vi "Autonomous Independent.vi"   [LabVIEW 2016]
doc: "This VI is called when autonomous begins, and will automatically be terminated when autonomous ends. You can carry out timed or sensor driven robot movement independently without needing to return to the caller."
uses:
  <vilib>/Rock Robotics/Network Tables/NT Read String.vi
panel:
  # "Be sure to right-click and choose Data Operations>>Make Current Value default if you want to save the array values with the VI"
types:
  T1 = typedef "WPI_MotorControlDeviceRef.ctl" = cluster{"DeviceStatus":errorcluster, "Type":T2, "PWM":cluster{"PWM Channel":T3, "DeadBand":T4}, "CAN":cluster{"Device Number":u8, "SetOutput VI Ref":variant, "GetOutput VI Ref":variant, "Enable VI Ref":variant, "Disable VI Ref":variant, "Data":variant}, "Invert":bool}
  T2 = typedef "WPI_MotorControlType.ctl" = enum16{"PWM", "CAN"}
  T3 = typedef "FPGA_DIOPWMChannel.ctl" = enum8{"PWM 0", "PWM 1", "PWM 2", "PWM 3", "PWM 4", "PWM 5", "PWM 6", "PWM 7", "PWM 8", "PWM 9", "PWM MXP 0", "PWM MXP 1", "PWM MXP 2", "PWM MXP 3", "PWM MXP 4", "PWM MXP 5", "PWM MXP 6", "PWM MXP 7", "PWM MXP 8", "PWM MXP 9", "Invalid"}
  T4 = typedef "WPI_PWMDeadband.ctl" = cluster{"Name":string, "maxPositivePwm":i32, "minPositivePwm":i32, "centerPwm":i32, "maxNegativePwm":i32, "minNegativePwm":i32, "angularRange":u16}
  T5 = typedef "WPI_DriverStationAllianceInfo.ctl" = enum16{"Red", "Blue", "Invalid"}
  T6 = typedef "WPI_EncoderDevRef.ctl" = cluster{"DevStatus":errorcluster, "EncoderIndex":T7, "CounterIndex":T8, "DistancePerCount":dbl, "Decoding Type":T9}
  T7 = typedef "FPGA_EncoderIdx.ctl" = enum8{"Enc 0", "Enc 1", "Enc 2", "Enc 3", "Enc 4", "Enc 5", "Enc 6", "Enc 7", "Invalid"}
  T8 = typedef "FPGA_CounterCtrSystemIndex.ctl" = enum8{"Ctr 0", "Ctr 1", "Ctr 2", "Ctr 3", "Ctr 4", "Ctr 5", "Ctr 6", "Ctr 7", "Invalid"}
  T9 = typedef "WPI_EncoderType.ctl" = enum16{"1x", "2x", "4x"}
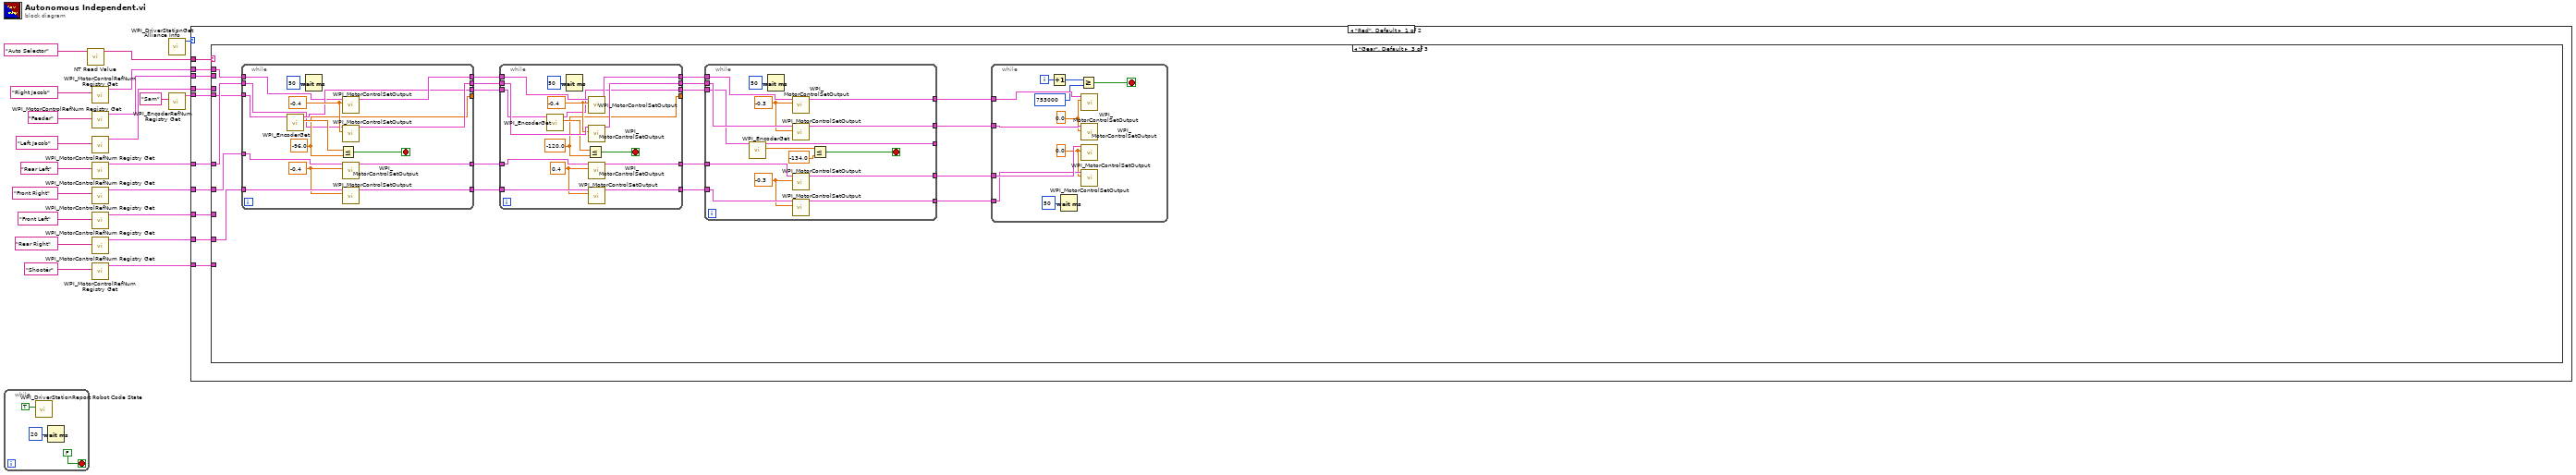
[diagram p0: block diagram]
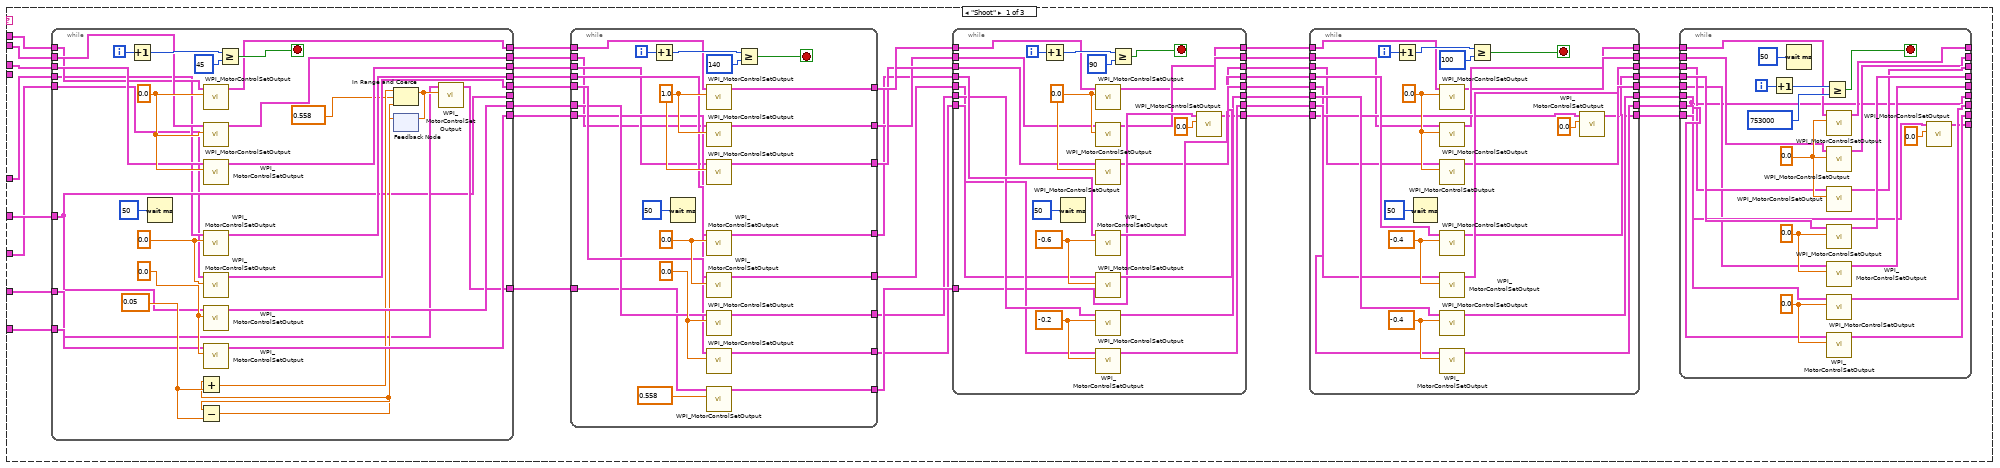
[diagram p2: hidden frame]
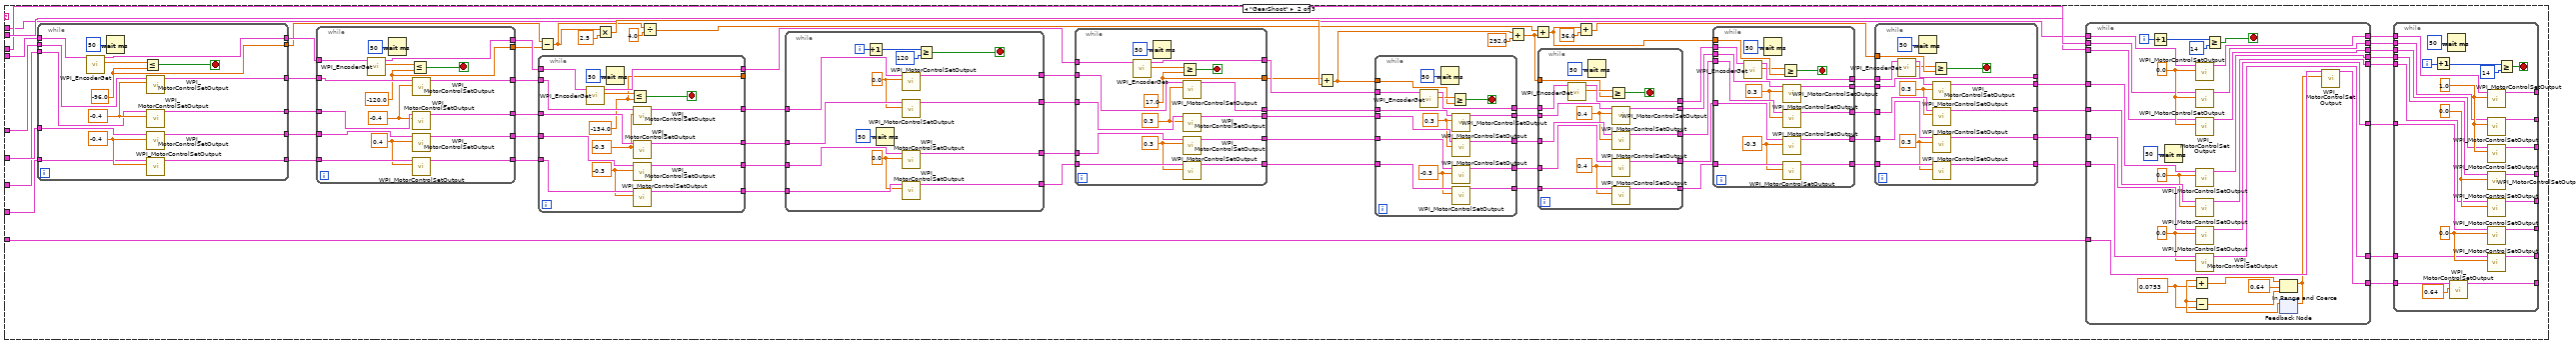
[diagram p3: hidden frame]
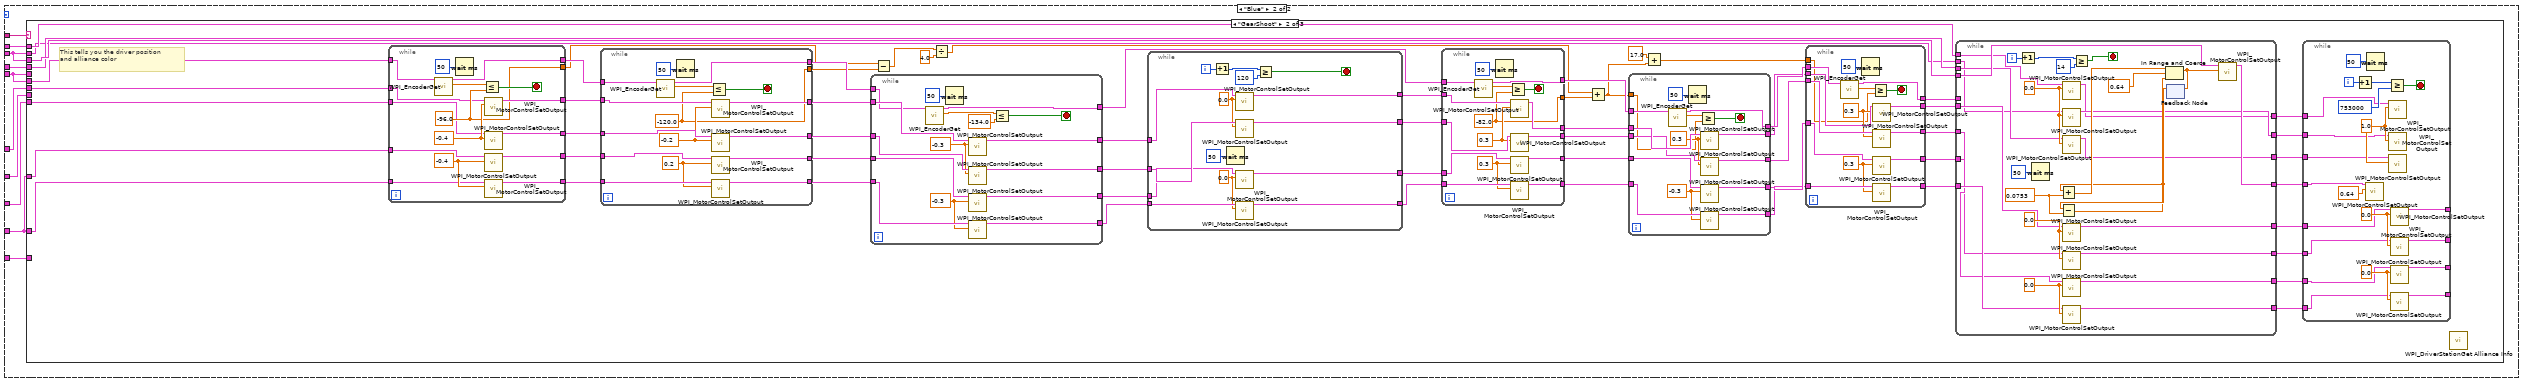
[diagram p4: hidden frame]
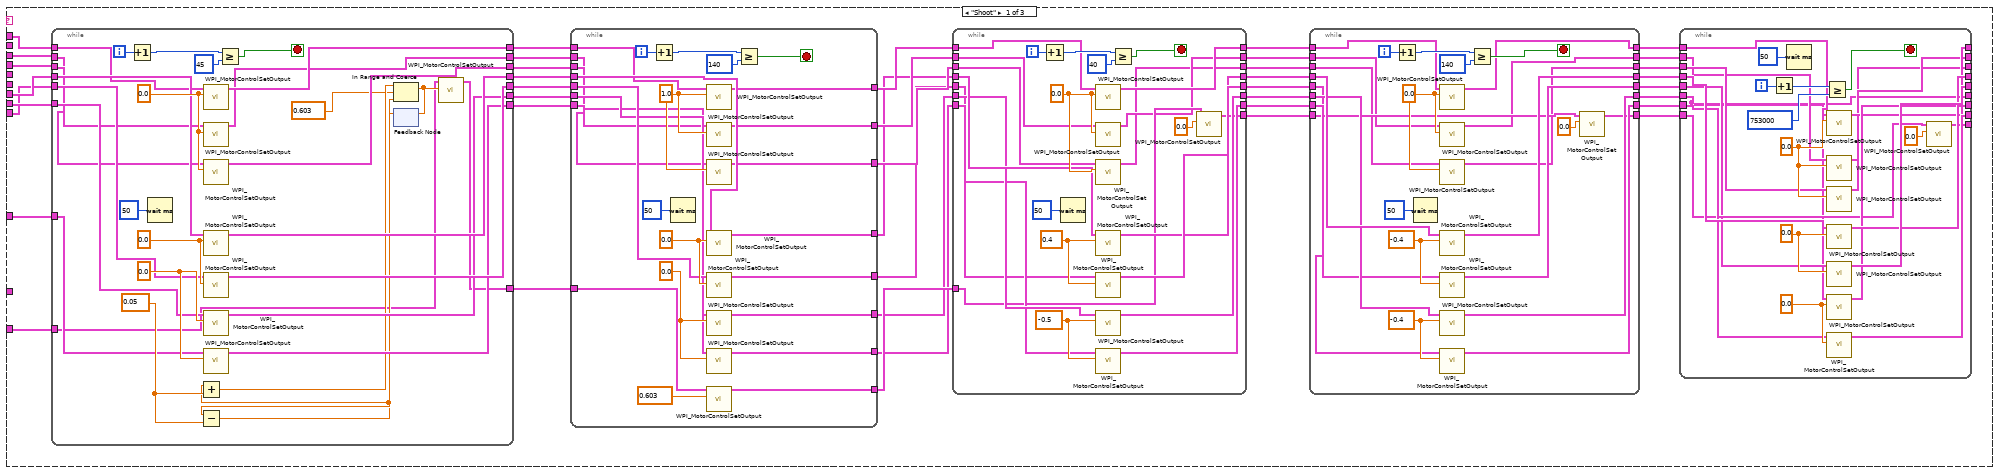
[diagram p5: hidden frame]
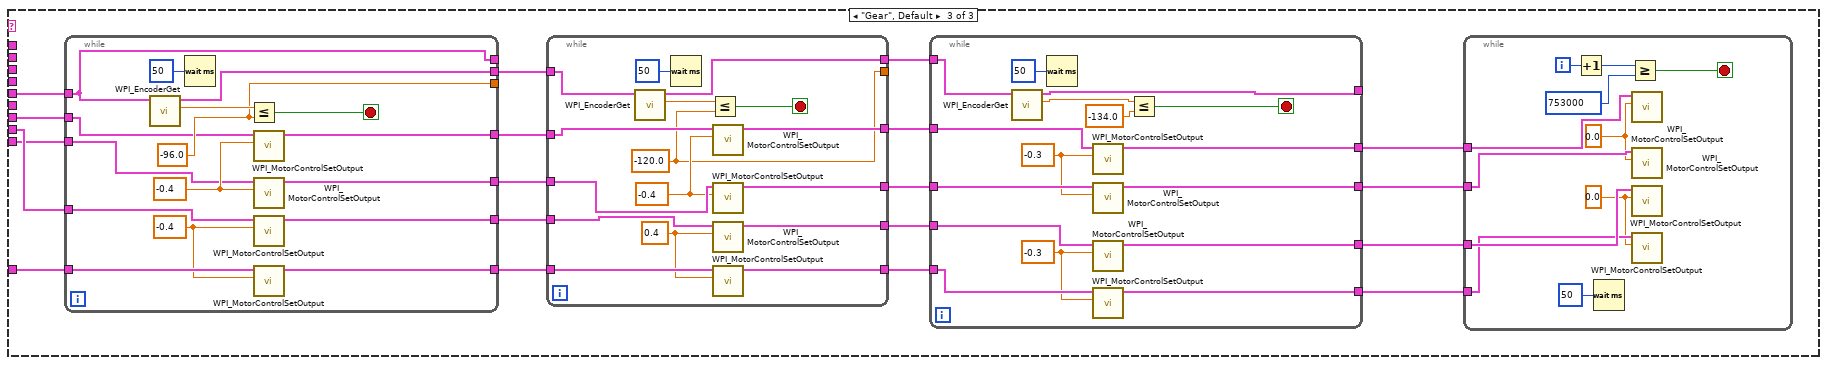
[diagram p6: hidden frame]
diagram:
  n1 = while {
    stop <- FALSE stop-if-true
    n2 = call <vilib>:"WPI_DriverStationReport Robot Code State.vi"("Autonomous"=TRUE) -> ()  [unwired: 10 in, 1 out]
    n3 = Wait (ms)(milliseconds to wait=u32 20) -> ()  [unwired: 1 out]
  }
  n4 = call-poly <vilib>:"NT Read Value.vi"("Name"="Auto Selector") -> ("String"=w1:string)  [unwired: 9 in, 1 out]
  n5 = call <vilib>:"WPI_MotorControlRefNum Registry Get.vi"("refnum name"="Right Jacob") -> ("MotorControlDevRef"=w8:T1)  [unwired: 9 in, 1 out]
  n6 = call <vilib>:"WPI_MotorControlRefNum Registry Get.vi"("refnum name"="Feeder") -> ("MotorControlDevRef"=w4:T1)  [unwired: 9 in, 1 out]
  n7 = call <vilib>:"WPI_MotorControlRefNum Registry Get.vi"("refnum name"="Left Jacob") -> ("MotorControlDevRef"=w3:T1)  [unwired: 9 in, 1 out]
  n8 = call <vilib>:"WPI_MotorControlRefNum Registry Get.vi"("refnum name"="Rear Left") -> ("MotorControlDevRef"=w7:T1)  [unwired: 9 in, 1 out]
  n9 = call <vilib>:"WPI_MotorControlRefNum Registry Get.vi"("refnum name"="Front Right") -> ("MotorControlDevRef"=w9:T1)  [unwired: 9 in, 1 out]
  n10 = call <vilib>:"WPI_MotorControlRefNum Registry Get.vi"("refnum name"="Front Left") -> ("MotorControlDevRef"=w2:T1)  [unwired: 9 in, 1 out]
  n11 = call <vilib>:"WPI_MotorControlRefNum Registry Get.vi"("refnum name"="Rear Right") -> ("MotorControlDevRef"=w10:T1)  [unwired: 9 in, 1 out]
  n12 = call <vilib>:"WPI_MotorControlRefNum Registry Get.vi"("refnum name"="Shootér") -> ("MotorControlDevRef"=w5:T1)  [unwired: 9 in, 1 out]
  n13 = call <vilib>:"WPI_DriverStationGet Alliance Info.vi"() -> ("Alliance"=w20:T5)  [unwired: 11 out]
  n14 = call <vilib>:"WPI_EncoderRefNum Registry Get.vi"("refnum name"="Sam") -> ("EncoderDevRef"=w6:T6)  [unwired: 9 in, 1 out]
  n15 = case shown="\"Red\", Default" w20 {
    tunnel: w10 -> [w34 w557]
    tunnel: w9 -> [w33 w563]
    tunnel: w8 -> [w32 w559]
    tunnel: w7 -> [w31 w562]
    tunnel: w6 -> [w30 w556]
    tunnel: w5 -> [w29 w558]
    tunnel: w4 -> [w28 w555]
    tunnel: w3 -> [w27 w560]
    tunnel: w2 -> [w26 w561]
    tunnel: w1 -> [w25 w564]
    frame "Red", Default {
      n16 = case shown="\"Gear\", Default" w25 {
        tunnel: w34 -> [w38 w208 w481]
        tunnel: w33 -> [w37 w207 w480]
        tunnel: w32 -> [w39 w211 w479]
        tunnel: w31 -> [w36 w206 w478]
        tunnel: w30 -> [_ w209 w477]
        tunnel: w29 -> [w42 w210 _]
        tunnel: w28 -> [w41 w213 _]
        tunnel: w27 -> [w40 w212 _]
        tunnel: w26 -> [w35 w205 _]
        frame "Shoot" {
          n17 = while {
            tunnel: [w177] -> w73
            tunnel: [w176] -> w74
            tunnel: [w174] -> w72
            tunnel: [w173] -> w71
            tunnel: [w165] -> w70
            tunnel: [w164] -> w69
            tunnel: [w163] -> w68
            tunnel: [w162] -> w67
            tunnel: w42 -> [w157]
            tunnel: w41 -> [w156]
            tunnel: w40 -> [w155]
            tunnel: w39 -> [w154]
            tunnel: w38 -> [w153]
            tunnel: [w152] -> _
            tunnel: w37 -> [w152]
            tunnel: w36 -> [w151]
            tunnel: w35 -> [w150]
            i -> [w172]
            stop <- w169 stop-if-true
            w166 = 0.05
            w168 = 0.0 ("Output")
            w175 = 0.0 ("Output")
            w178 = 0.0 ("Output")
            n18 = Increment(x=w172) -> (x+1=w171:i32)
            n19 = Wait (ms)(milliseconds to wait=u32 50) -> ()  [unwired: 1 out]
            n20 = call <vilib>:"WPI_MotorControlSetOutput.vi"("Output"=w168, "MotorControlDevRef"=w154) -> ("MotorControlDevRef"=w164:T1)  [unwired: 7 in, 2 out]
            n21 = call <vilib>:"WPI_MotorControlSetOutput.vi"("Output"=w168, "MotorControlDevRef"=w156) -> ("MotorControlDevRef"=w162:T1)  [unwired: 7 in, 2 out]
            n22 = call <vilib>:"WPI_MotorControlSetOutput.vi"("Output"=w168, "MotorControlDevRef"=w155) -> ("MotorControlDevRef"=w163:T1)  [unwired: 7 in, 2 out]
            n23 = call <vilib>:"WPI_MotorControlSetOutput.vi"("Output"=w178, "MotorControlDevRef"=w151) -> ("MotorControlDevRef"=w176:T1)  [unwired: 7 in, 2 out]
            n24 = call <vilib>:"WPI_MotorControlSetOutput.vi"("Output"=w178, "MotorControlDevRef"=w150) -> ("MotorControlDevRef"=w177:T1)  [unwired: 7 in, 2 out]
            n25 = call <vilib>:"WPI_MotorControlSetOutput.vi"("Output"=w175, "MotorControlDevRef"=w152) -> ("MotorControlDevRef"=w174:T1)  [unwired: 7 in, 2 out]
            n26 = call <vilib>:"WPI_MotorControlSetOutput.vi"("Output"=w175, "MotorControlDevRef"=w153) -> ("MotorControlDevRef"=w173:T1)  [unwired: 7 in, 2 out]
            n27 = Greater Or Equal?(x=w171, y=45) -> (x >= y?=w169:bool)
            n28 = feedback #1() -> (w160:dbl)  [unwired: 1 in]
            n29 = Add(x=w160, y=w166) -> (x+y=w167:dbl)
            n30 = Subtract(x=w160, y=w166) -> (x-y=w158:dbl)
            n31 = In Range and Coerce(upper limit=w167, x=0.558 ("Output"), lower limit=w158) -> (coerced(x)=w161:dbl)  [unwired: 1 out]
            n32 = feedback-in #1(w161) -> ()
            n33 = call <vilib>:"WPI_MotorControlSetOutput.vi"("Output"=w161, "MotorControlDevRef"=w157) -> ("MotorControlDevRef"=w165:T1)  [unwired: 7 in, 2 out]
          }
          n34 = while {
            tunnel: [w202] -> w60
            tunnel: [w201] -> w59
            tunnel: [w199] -> w62
            tunnel: [w198] -> w61
            tunnel: w74 -> [w191]
            tunnel: w73 -> [w190]
            tunnel: w72 -> [w189]
            tunnel: w71 -> [w188]
            tunnel: w70 -> [w187]
            tunnel: w69 -> [w186]
            tunnel: w68 -> [w185]
            tunnel: w67 -> [w184]
            tunnel: [w183] -> w64
            tunnel: [w182] -> w63
            tunnel: [w181] -> w65
            tunnel: [w180] -> w66
            i -> [w197]
            stop <- w194 stop-if-true
            w193 = 1.0 ("Output")
            w200 = 0.0 ("Output")
            w203 = 0.0 ("Output")
            n35 = Increment(x=w197) -> (x+1=w196:i32)
            n36 = Wait (ms)(milliseconds to wait=u32 50) -> ()  [unwired: 1 out]
            n37 = call <vilib>:"WPI_MotorControlSetOutput.vi"("Output"=w193, "MotorControlDevRef"=w186) -> ("MotorControlDevRef"=w181:T1)  [unwired: 7 in, 2 out]
            n38 = call <vilib>:"WPI_MotorControlSetOutput.vi"("Output"=w193, "MotorControlDevRef"=w184) -> ("MotorControlDevRef"=w182:T1)  [unwired: 7 in, 2 out]
            n39 = call <vilib>:"WPI_MotorControlSetOutput.vi"("Output"=w193, "MotorControlDevRef"=w185) -> ("MotorControlDevRef"=w183:T1)  [unwired: 7 in, 2 out]
            n40 = call <vilib>:"WPI_MotorControlSetOutput.vi"("Output"=w203, "MotorControlDevRef"=w191) -> ("MotorControlDevRef"=w201:T1)  [unwired: 7 in, 2 out]
            n41 = call <vilib>:"WPI_MotorControlSetOutput.vi"("Output"=w203, "MotorControlDevRef"=w190) -> ("MotorControlDevRef"=w202:T1)  [unwired: 7 in, 2 out]
            n42 = call <vilib>:"WPI_MotorControlSetOutput.vi"("Output"=w200, "MotorControlDevRef"=w189) -> ("MotorControlDevRef"=w199:T1)  [unwired: 7 in, 2 out]
            n43 = call <vilib>:"WPI_MotorControlSetOutput.vi"("Output"=w200, "MotorControlDevRef"=w188) -> ("MotorControlDevRef"=w198:T1)  [unwired: 7 in, 2 out]
            n44 = call <vilib>:"WPI_MotorControlSetOutput.vi"("Output"=0.558, "MotorControlDevRef"=w187) -> ("MotorControlDevRef"=w180:T1)  [unwired: 7 in, 2 out]
            n45 = Greater Or Equal?(x=w196, y=140) -> (x >= y?=w194:bool)
          }
          n46 = while {
            tunnel: [w147] -> w52
            tunnel: [w146] -> w51
            tunnel: [w144] -> w54
            tunnel: [w143] -> w53
            tunnel: w59 -> [w136]
            tunnel: w62 -> [w135]
            tunnel: w61 -> [w134]
            tunnel: w66 -> [w133]
            tunnel: w65 -> [w132]
            tunnel: w64 -> [w131]
            tunnel: w63 -> [w130]
            tunnel: [w129] -> w56
            tunnel: [w128] -> w55
            tunnel: [w127] -> w57
            tunnel: [w126] -> w58
            tunnel: w60 -> [w125]
            i -> [w142]
            stop <- w139 stop-if-true
            w138 = 0.0 ("Output")
            w145 = -0.2 ("Output")
            w148 = -0.6 ("Output")
            n47 = Increment(x=w142) -> (x+1=w141:i32)
            n48 = Wait (ms)(milliseconds to wait=u32 50) -> ()  [unwired: 1 out]
            n49 = call <vilib>:"WPI_MotorControlSetOutput.vi"("Output"=w138, "MotorControlDevRef"=w132) -> ("MotorControlDevRef"=w127:T1)  [unwired: 7 in, 2 out]
            n50 = call <vilib>:"WPI_MotorControlSetOutput.vi"("Output"=w138, "MotorControlDevRef"=w130) -> ("MotorControlDevRef"=w128:T1)  [unwired: 7 in, 2 out]
            n51 = call <vilib>:"WPI_MotorControlSetOutput.vi"("Output"=w138, "MotorControlDevRef"=w131) -> ("MotorControlDevRef"=w129:T1)  [unwired: 7 in, 2 out]
            n52 = call <vilib>:"WPI_MotorControlSetOutput.vi"("Output"=w148, "MotorControlDevRef"=w136) -> ("MotorControlDevRef"=w146:T1)  [unwired: 7 in, 2 out]
            n53 = call <vilib>:"WPI_MotorControlSetOutput.vi"("Output"=w148, "MotorControlDevRef"=w125) -> ("MotorControlDevRef"=w147:T1)  [unwired: 7 in, 2 out]
            n54 = call <vilib>:"WPI_MotorControlSetOutput.vi"("Output"=w145, "MotorControlDevRef"=w135) -> ("MotorControlDevRef"=w144:T1)  [unwired: 7 in, 2 out]
            n55 = call <vilib>:"WPI_MotorControlSetOutput.vi"("Output"=w145, "MotorControlDevRef"=w134) -> ("MotorControlDevRef"=w143:T1)  [unwired: 7 in, 2 out]
            n56 = Greater Or Equal?(x=w141, y=90) -> (x >= y?=w139:bool)
            n57 = call <vilib>:"WPI_MotorControlSetOutput.vi"("Output"=0.0, "MotorControlDevRef"=w133) -> ("MotorControlDevRef"=w126:T1)  [unwired: 7 in, 2 out]
          }
          n58 = while {
            tunnel: [w122] -> w44
            tunnel: [w121] -> w43
            tunnel: [w119] -> w46
            tunnel: [w118] -> w45
            tunnel: w51 -> [w111]
            tunnel: w54 -> [w110]
            tunnel: w53 -> [w109]
            tunnel: w58 -> [w108]
            tunnel: w57 -> [w107]
            tunnel: w56 -> [w106]
            tunnel: w55 -> [w105]
            tunnel: [w104] -> w48
            tunnel: [w103] -> w47
            tunnel: [w102] -> w49
            tunnel: [w101] -> w50
            tunnel: w52 -> [w100]
            i -> [w117]
            stop <- w114 stop-if-true
            w113 = 0.0 ("Output")
            w120 = -0.4 ("Output")
            w123 = -0.4 ("Output")
            n59 = Increment(x=w117) -> (x+1=w116:i32)
            n60 = Wait (ms)(milliseconds to wait=u32 50) -> ()  [unwired: 1 out]
            n61 = call <vilib>:"WPI_MotorControlSetOutput.vi"("Output"=w113, "MotorControlDevRef"=w107) -> ("MotorControlDevRef"=w102:T1)  [unwired: 7 in, 2 out]
            n62 = call <vilib>:"WPI_MotorControlSetOutput.vi"("Output"=w113, "MotorControlDevRef"=w105) -> ("MotorControlDevRef"=w103:T1)  [unwired: 7 in, 2 out]
            n63 = call <vilib>:"WPI_MotorControlSetOutput.vi"("Output"=w113, "MotorControlDevRef"=w106) -> ("MotorControlDevRef"=w104:T1)  [unwired: 7 in, 2 out]
            n64 = call <vilib>:"WPI_MotorControlSetOutput.vi"("Output"=w123, "MotorControlDevRef"=w111) -> ("MotorControlDevRef"=w121:T1)  [unwired: 7 in, 2 out]
            n65 = call <vilib>:"WPI_MotorControlSetOutput.vi"("Output"=w123, "MotorControlDevRef"=w100) -> ("MotorControlDevRef"=w122:T1)  [unwired: 7 in, 2 out]
            n66 = call <vilib>:"WPI_MotorControlSetOutput.vi"("Output"=w120, "MotorControlDevRef"=w110) -> ("MotorControlDevRef"=w119:T1)  [unwired: 7 in, 2 out]
            n67 = call <vilib>:"WPI_MotorControlSetOutput.vi"("Output"=w120, "MotorControlDevRef"=w109) -> ("MotorControlDevRef"=w118:T1)  [unwired: 7 in, 2 out]
            n68 = Greater Or Equal?(x=w116, y=100) -> (x >= y?=w114:bool)
            n69 = call <vilib>:"WPI_MotorControlSetOutput.vi"("Output"=0.0, "MotorControlDevRef"=w108) -> ("MotorControlDevRef"=w101:T1)  [unwired: 7 in, 2 out]
          }
          n70 = while {
            tunnel: [w97] -> _
            tunnel: [w96] -> _
            tunnel: [w94] -> _
            tunnel: [w93] -> _
            tunnel: w43 -> [w86]
            tunnel: w46 -> [w75]
            tunnel: w45 -> [w85]
            tunnel: w50 -> [w84]
            tunnel: w49 -> [w83]
            tunnel: w48 -> [w82]
            tunnel: w47 -> [w81]
            tunnel: [w80] -> _
            tunnel: [w79] -> _
            tunnel: [w78] -> _
            tunnel: [w77] -> _
            tunnel: w44 -> [w76]
            tunnel: [w75] -> _
            i -> [w92]
            stop <- w89 stop-if-true
            w88 = 0.0 ("Output")
            w95 = 0.0 ("Output")
            w98 = 0.0 ("Output")
            n71 = Increment(x=w92) -> (x+1=w91:i32)
            n72 = Wait (ms)(milliseconds to wait=u32 50) -> ()  [unwired: 1 out]
            n73 = Greater Or Equal?(x=w91, y=753000) -> (x >= y?=w89:bool)
            n74 = call <vilib>:"WPI_MotorControlSetOutput.vi"("Output"=w88, "MotorControlDevRef"=w83) -> ("MotorControlDevRef"=w78:T1)  [unwired: 7 in, 2 out]
            n75 = call <vilib>:"WPI_MotorControlSetOutput.vi"("Output"=w88, "MotorControlDevRef"=w81) -> ("MotorControlDevRef"=w79:T1)  [unwired: 7 in, 2 out]
            n76 = call <vilib>:"WPI_MotorControlSetOutput.vi"("Output"=w88, "MotorControlDevRef"=w82) -> ("MotorControlDevRef"=w80:T1)  [unwired: 7 in, 2 out]
            n77 = call <vilib>:"WPI_MotorControlSetOutput.vi"("Output"=w98, "MotorControlDevRef"=w86) -> ("MotorControlDevRef"=w96:T1)  [unwired: 7 in, 2 out]
            n78 = call <vilib>:"WPI_MotorControlSetOutput.vi"("Output"=w98, "MotorControlDevRef"=w76) -> ("MotorControlDevRef"=w97:T1)  [unwired: 7 in, 2 out]
            n79 = call <vilib>:"WPI_MotorControlSetOutput.vi"("Output"=w95, "MotorControlDevRef"=w75) -> ("MotorControlDevRef"=w94:T1)  [unwired: 7 in, 2 out]
            n80 = call <vilib>:"WPI_MotorControlSetOutput.vi"("Output"=w95, "MotorControlDevRef"=w85) -> ("MotorControlDevRef"=w93:T1)  [unwired: 7 in, 2 out]
            n81 = call <vilib>:"WPI_MotorControlSetOutput.vi"("Output"=0.0, "MotorControlDevRef"=w84) -> ("MotorControlDevRef"=w77:T1)  [unwired: 7 in, 2 out]
          }
        }
        frame "GearShoot" {
          n82 = while {
            tunnel: [w474] -> w277
            tunnel: [w473] -> w278
            tunnel: [w471] -> w276
            tunnel: [w470] -> w275
            tunnel: [w467] -> w269
            tunnel: [w466] -> w239
            tunnel: w209 -> [w465]
            tunnel: w208 -> [w464]
            tunnel: w207 -> [w463]
            tunnel: w206 -> [w462]
            tunnel: w205 -> [w461]
            stop <- w468 stop-if-true
            w466 = -96.0 ("y")
            w472 = -0.4 ("Output")
            w475 = -0.4 ("Output")
            n83 = call <vilib>:"WPI_EncoderGet.vi"("EncoderDevRef"=w465) -> ("Distance"=w469:dbl, "EncoderDevRef"=w467:T6)  [unwired: 5 in, 4 out]
            n84 = Wait (ms)(milliseconds to wait=u32 50) -> ()  [unwired: 1 out]
            n85 = Less Or Equal?(x=w469, y=w466) -> (x <= y?=w468:bool)
            n86 = call <vilib>:"WPI_MotorControlSetOutput.vi"("Output"=w475, "MotorControlDevRef"=w462) -> ("MotorControlDevRef"=w473:T1)  [unwired: 7 in, 2 out]
            n87 = call <vilib>:"WPI_MotorControlSetOutput.vi"("Output"=w475, "MotorControlDevRef"=w461) -> ("MotorControlDevRef"=w474:T1)  [unwired: 7 in, 2 out]
            n88 = call <vilib>:"WPI_MotorControlSetOutput.vi"("Output"=w472, "MotorControlDevRef"=w463) -> ("MotorControlDevRef"=w471:T1)  [unwired: 7 in, 2 out]
            n89 = call <vilib>:"WPI_MotorControlSetOutput.vi"("Output"=w472, "MotorControlDevRef"=w464) -> ("MotorControlDevRef"=w470:T1)  [unwired: 7 in, 2 out]
          }
          n90 = while {
            tunnel: w278 -> [w459]
            tunnel: w277 -> [w458]
            tunnel: [w456] -> w273
            tunnel: [w455] -> w274
            tunnel: w276 -> [w454]
            tunnel: w275 -> [w453]
            tunnel: [w451] -> w272
            tunnel: [w450] -> w271
            tunnel: [w447] -> w270
            tunnel: w269 -> [w446]
            tunnel: [w445] -> w238
            stop <- w448 stop-if-true
            w445 = -120.0 ("y")
            w452 = 0.4 ("Output")
            w457 = -0.4 ("Output")
            n91 = call <vilib>:"WPI_EncoderGet.vi"("EncoderDevRef"=w446) -> ("Distance"=w449:dbl, "EncoderDevRef"=w447:T6)  [unwired: 5 in, 4 out]
            n92 = Wait (ms)(milliseconds to wait=u32 50) -> ()  [unwired: 1 out]
            n93 = Less Or Equal?(x=w449, y=w445) -> (x <= y?=w448:bool)
            n94 = call <vilib>:"WPI_MotorControlSetOutput.vi"("Output"=w457, "MotorControlDevRef"=w459) -> ("MotorControlDevRef"=w455:T1)  [unwired: 7 in, 2 out]
            n95 = call <vilib>:"WPI_MotorControlSetOutput.vi"("Output"=w457, "MotorControlDevRef"=w458) -> ("MotorControlDevRef"=w456:T1)  [unwired: 7 in, 2 out]
            n96 = call <vilib>:"WPI_MotorControlSetOutput.vi"("Output"=w452, "MotorControlDevRef"=w454) -> ("MotorControlDevRef"=w451:T1)  [unwired: 7 in, 2 out]
            n97 = call <vilib>:"WPI_MotorControlSetOutput.vi"("Output"=w452, "MotorControlDevRef"=w453) -> ("MotorControlDevRef"=w450:T1)  [unwired: 7 in, 2 out]
          }
          n98 = Subtract(x=w239, y=w238) -> (x-y=w229:dbl)
          n99 = while {
            tunnel: w274 -> [w443]
            tunnel: w273 -> [w442]
            tunnel: [w440] -> w267
            tunnel: [w439] -> w268
            tunnel: w272 -> [w438]
            tunnel: w271 -> [w437]
            tunnel: [w435] -> w266
            tunnel: [w434] -> w265
            tunnel: [w431] -> w240
            tunnel: w270 -> [w430]
            tunnel: [w429] -> _
            stop <- w432 stop-if-true
            w429 = -134.0 ("y")
            w436 = -0.3 ("Output")
            w441 = -0.3 ("Output")
            n100 = call <vilib>:"WPI_EncoderGet.vi"("EncoderDevRef"=w430) -> ("Distance"=w433:dbl, "EncoderDevRef"=w431:T6)  [unwired: 5 in, 4 out]
            n101 = Wait (ms)(milliseconds to wait=u32 50) -> ()  [unwired: 1 out]
            n102 = Less Or Equal?(x=w433, y=w429) -> (x <= y?=w432:bool)
            n103 = call <vilib>:"WPI_MotorControlSetOutput.vi"("Output"=w441, "MotorControlDevRef"=w443) -> ("MotorControlDevRef"=w439:T1)  [unwired: 7 in, 2 out]
            n104 = call <vilib>:"WPI_MotorControlSetOutput.vi"("Output"=w441, "MotorControlDevRef"=w442) -> ("MotorControlDevRef"=w440:T1)  [unwired: 7 in, 2 out]
            n105 = call <vilib>:"WPI_MotorControlSetOutput.vi"("Output"=w436, "MotorControlDevRef"=w438) -> ("MotorControlDevRef"=w435:T1)  [unwired: 7 in, 2 out]
            n106 = call <vilib>:"WPI_MotorControlSetOutput.vi"("Output"=w436, "MotorControlDevRef"=w437) -> ("MotorControlDevRef"=w434:T1)  [unwired: 7 in, 2 out]
          }
          n107 = Multiply(x=w229, y=2.5) -> (x*y=w236:dbl)
          n108 = Divide(x=w229, y=4.0) -> (x/y=w231:dbl)
          n109 = while {
            tunnel: w268 -> [w427]
            tunnel: w267 -> [w426]
            tunnel: [w424] -> w246
            tunnel: [w423] -> w247
            tunnel: w266 -> [w422]
            tunnel: w265 -> [w421]
            tunnel: [w419] -> w245
            tunnel: [w418] -> w244
            i -> [w417]
            stop <- w414 stop-if-true
            w420 = 0.0 ("Output")
            w425 = 0.0 ("Output")
            n110 = Increment(x=w417) -> (x+1=w416:i32)
            n111 = Wait (ms)(milliseconds to wait=u32 50) -> ()  [unwired: 1 out]
            n112 = call <vilib>:"WPI_MotorControlSetOutput.vi"("Output"=w425, "MotorControlDevRef"=w427) -> ("MotorControlDevRef"=w423:T1)  [unwired: 7 in, 2 out]
            n113 = call <vilib>:"WPI_MotorControlSetOutput.vi"("Output"=w425, "MotorControlDevRef"=w426) -> ("MotorControlDevRef"=w424:T1)  [unwired: 7 in, 2 out]
            n114 = call <vilib>:"WPI_MotorControlSetOutput.vi"("Output"=w420, "MotorControlDevRef"=w422) -> ("MotorControlDevRef"=w419:T1)  [unwired: 7 in, 2 out]
            n115 = call <vilib>:"WPI_MotorControlSetOutput.vi"("Output"=w420, "MotorControlDevRef"=w421) -> ("MotorControlDevRef"=w418:T1)  [unwired: 7 in, 2 out]
            n116 = Greater Or Equal?(x=w416, y=120) -> (x >= y?=w414:bool)
          }
          n117 = while {
            tunnel: w247 -> [w412]
            tunnel: w246 -> [w411]
            tunnel: [w409] -> w254
            tunnel: [w408] -> w255
            tunnel: w245 -> [w407]
            tunnel: w244 -> [w406]
            tunnel: [w404] -> w253
            tunnel: [w403] -> w252
            tunnel: [w402] -> w241
            tunnel: w240 -> [w401]
            tunnel: [w398] -> w234
            stop <- w399 stop-if-true
            w398 = 17.0 ("y")
            w405 = 0.3 ("Output")
            w410 = 0.3 ("Output")
            n118 = call <vilib>:"WPI_EncoderGet.vi"("EncoderDevRef"=w401) -> ("Distance"=w400:dbl, "EncoderDevRef"=w402:T6)  [unwired: 5 in, 4 out]
            n119 = Wait (ms)(milliseconds to wait=u32 50) -> ()  [unwired: 1 out]
            n120 = Greater Or Equal?(x=w400, y=w398) -> (x >= y?=w399:bool)
            n121 = call <vilib>:"WPI_MotorControlSetOutput.vi"("Output"=w410, "MotorControlDevRef"=w412) -> ("MotorControlDevRef"=w408:T1)  [unwired: 7 in, 2 out]
            n122 = call <vilib>:"WPI_MotorControlSetOutput.vi"("Output"=w410, "MotorControlDevRef"=w411) -> ("MotorControlDevRef"=w409:T1)  [unwired: 7 in, 2 out]
            n123 = call <vilib>:"WPI_MotorControlSetOutput.vi"("Output"=w405, "MotorControlDevRef"=w407) -> ("MotorControlDevRef"=w404:T1)  [unwired: 7 in, 2 out]
            n124 = call <vilib>:"WPI_MotorControlSetOutput.vi"("Output"=w405, "MotorControlDevRef"=w406) -> ("MotorControlDevRef"=w403:T1)  [unwired: 7 in, 2 out]
          }
          n125 = Add(x=w234, y=w236) -> (x+y=w233:dbl)
          n126 = while {
            tunnel: w255 -> [w396]
            tunnel: w254 -> [w395]
            tunnel: [w393] -> w250
            tunnel: [w392] -> w251
            tunnel: w253 -> [w391]
            tunnel: w252 -> [w390]
            tunnel: [w388] -> w249
            tunnel: [w387] -> w248
            tunnel: [w386] -> w242
            tunnel: w241 -> [w385]
            tunnel: w233 -> [w382]
            stop <- w383 stop-if-true
            w389 = -0.3 ("Output")
            w394 = 0.3 ("Output")
            n127 = call <vilib>:"WPI_EncoderGet.vi"("EncoderDevRef"=w385) -> ("Distance"=w384:dbl, "EncoderDevRef"=w386:T6)  [unwired: 5 in, 4 out]
            n128 = Wait (ms)(milliseconds to wait=u32 50) -> ()  [unwired: 1 out]
            n129 = Greater Or Equal?(x=w384, y=w382) -> (x >= y?=w383:bool)
            n130 = call <vilib>:"WPI_MotorControlSetOutput.vi"("Output"=w394, "MotorControlDevRef"=w396) -> ("MotorControlDevRef"=w392:T1)  [unwired: 7 in, 2 out]
            n131 = call <vilib>:"WPI_MotorControlSetOutput.vi"("Output"=w394, "MotorControlDevRef"=w395) -> ("MotorControlDevRef"=w393:T1)  [unwired: 7 in, 2 out]
            n132 = call <vilib>:"WPI_MotorControlSetOutput.vi"("Output"=w389, "MotorControlDevRef"=w391) -> ("MotorControlDevRef"=w388:T1)  [unwired: 7 in, 2 out]
            n133 = call <vilib>:"WPI_MotorControlSetOutput.vi"("Output"=w389, "MotorControlDevRef"=w390) -> ("MotorControlDevRef"=w387:T1)  [unwired: 7 in, 2 out]
          }
          n134 = Add(x=w233, y=292.0) -> (x+y=w230:dbl)
          n135 = Add(x=w231, y=w230) -> (x+y=w227:dbl)
          n136 = while {
            tunnel: w251 -> [w380]
            tunnel: w250 -> [w379]
            tunnel: [w377] -> w258
            tunnel: [w376] -> w259
            tunnel: w249 -> [w375]
            tunnel: w248 -> [w374]
            tunnel: [w372] -> w257
            tunnel: [w371] -> w256
            tunnel: [w370] -> w243
            tunnel: w242 -> [w369]
            tunnel: w230 -> [w367]
            stop <- w366 stop-if-true
            w373 = 0.4 ("Output")
            w378 = 0.4 ("Output")
            n137 = call <vilib>:"WPI_EncoderGet.vi"("EncoderDevRef"=w369) -> ("Distance"=w368:dbl, "EncoderDevRef"=w370:T6)  [unwired: 5 in, 4 out]
            n138 = Wait (ms)(milliseconds to wait=u32 50) -> ()  [unwired: 1 out]
            n139 = Greater Or Equal?(x=w368, y=w367) -> (x >= y?=w366:bool)
            n140 = call <vilib>:"WPI_MotorControlSetOutput.vi"("Output"=w378, "MotorControlDevRef"=w380) -> ("MotorControlDevRef"=w376:T1)  [unwired: 7 in, 2 out]
            n141 = call <vilib>:"WPI_MotorControlSetOutput.vi"("Output"=w378, "MotorControlDevRef"=w379) -> ("MotorControlDevRef"=w377:T1)  [unwired: 7 in, 2 out]
            n142 = call <vilib>:"WPI_MotorControlSetOutput.vi"("Output"=w373, "MotorControlDevRef"=w375) -> ("MotorControlDevRef"=w372:T1)  [unwired: 7 in, 2 out]
            n143 = call <vilib>:"WPI_MotorControlSetOutput.vi"("Output"=w373, "MotorControlDevRef"=w374) -> ("MotorControlDevRef"=w371:T1)  [unwired: 7 in, 2 out]
          }
          n144 = Add(x=w227, y=36.0) -> (x+y=w226:dbl)
          n145 = while {
            tunnel: w259 -> [w364]
            tunnel: w258 -> [w363]
            tunnel: [w361] -> w261
            tunnel: [w360] -> w260
            tunnel: w257 -> [w359]
            tunnel: w256 -> [w358]
            tunnel: [w356] -> w262
            tunnel: [w355] -> w263
            tunnel: [w354] -> w264
            tunnel: w243 -> [w353]
            tunnel: w227 -> [w352]
            stop <- w350 stop-if-true
            w357 = -0.3 ("Output")
            w362 = 0.3 ("Output")
            n146 = call <vilib>:"WPI_EncoderGet.vi"("EncoderDevRef"=w353) -> ("Distance"=w351:dbl, "EncoderDevRef"=w354:T6)  [unwired: 5 in, 4 out]
            n147 = Wait (ms)(milliseconds to wait=u32 50) -> ()  [unwired: 1 out]
            n148 = Greater Or Equal?(x=w351, y=w352) -> (x >= y?=w350:bool)
            n149 = call <vilib>:"WPI_MotorControlSetOutput.vi"("Output"=w362, "MotorControlDevRef"=w364) -> ("MotorControlDevRef"=w360:T1)  [unwired: 7 in, 2 out]
            n150 = call <vilib>:"WPI_MotorControlSetOutput.vi"("Output"=w362, "MotorControlDevRef"=w363) -> ("MotorControlDevRef"=w361:T1)  [unwired: 7 in, 2 out]
            n151 = call <vilib>:"WPI_MotorControlSetOutput.vi"("Output"=w357, "MotorControlDevRef"=w359) -> ("MotorControlDevRef"=w356:T1)  [unwired: 7 in, 2 out]
            n152 = call <vilib>:"WPI_MotorControlSetOutput.vi"("Output"=w357, "MotorControlDevRef"=w358) -> ("MotorControlDevRef"=w355:T1)  [unwired: 7 in, 2 out]
          }
          n153 = while {
            tunnel: w260 -> [w348]
            tunnel: w261 -> [w347]
            tunnel: [w345] -> w224
            tunnel: [w344] -> w223
            tunnel: w262 -> [w343]
            tunnel: w263 -> [w342]
            tunnel: [w340] -> w225
            tunnel: [w339] -> w222
            tunnel: [w338] -> _
            tunnel: w264 -> [w337]
            tunnel: w226 -> [w336]
            stop <- w334 stop-if-true
            w341 = 0.3 ("Output")
            w346 = 0.3 ("Output")
            n154 = call <vilib>:"WPI_EncoderGet.vi"("EncoderDevRef"=w337) -> ("Distance"=w335:dbl, "EncoderDevRef"=w338:T6)  [unwired: 5 in, 4 out]
            n155 = Wait (ms)(milliseconds to wait=u32 50) -> ()  [unwired: 1 out]
            n156 = Greater Or Equal?(x=w335, y=w336) -> (x >= y?=w334:bool)
            n157 = call <vilib>:"WPI_MotorControlSetOutput.vi"("Output"=w346, "MotorControlDevRef"=w348) -> ("MotorControlDevRef"=w344:T1)  [unwired: 7 in, 2 out]
            n158 = call <vilib>:"WPI_MotorControlSetOutput.vi"("Output"=w346, "MotorControlDevRef"=w347) -> ("MotorControlDevRef"=w345:T1)  [unwired: 7 in, 2 out]
            n159 = call <vilib>:"WPI_MotorControlSetOutput.vi"("Output"=w341, "MotorControlDevRef"=w343) -> ("MotorControlDevRef"=w340:T1)  [unwired: 7 in, 2 out]
            n160 = call <vilib>:"WPI_MotorControlSetOutput.vi"("Output"=w341, "MotorControlDevRef"=w342) -> ("MotorControlDevRef"=w339:T1)  [unwired: 7 in, 2 out]
          }
          n161 = while {
            tunnel: w223 -> [w333]
            tunnel: w224 -> [w332]
            tunnel: [w330] -> w216
            tunnel: [w329] -> w217
            tunnel: w225 -> [w328]
            tunnel: w222 -> [w327]
            tunnel: [w325] -> w215
            tunnel: [w320] -> w214
            tunnel: w210 -> [w318]
            tunnel: [w317] -> w218
            tunnel: [w316] -> w220
            tunnel: [w315] -> w219
            tunnel: [w314] -> w221
            tunnel: w213 -> [w306]
            tunnel: w212 -> [w305]
            tunnel: w211 -> [w304]
            i -> [w322]
            stop <- w321 stop-if-true
            w307 = 0.0753 ("y")
            w319 = 0.0 ("Output")
            w326 = 0.0 ("Output")
            w331 = 0.0 ("Output")
            n162 = Increment(x=w322) -> (x+1=w324:i32)
            n163 = Wait (ms)(milliseconds to wait=u32 50) -> ()  [unwired: 1 out]
            n164 = call <vilib>:"WPI_MotorControlSetOutput.vi"("Output"=w319, "MotorControlDevRef"=w304) -> ("MotorControlDevRef"=w314:T1)  [unwired: 7 in, 2 out]
            n165 = call <vilib>:"WPI_MotorControlSetOutput.vi"("Output"=w319, "MotorControlDevRef"=w306) -> ("MotorControlDevRef"=w316:T1)  [unwired: 7 in, 2 out]
            n166 = call <vilib>:"WPI_MotorControlSetOutput.vi"("Output"=w319, "MotorControlDevRef"=w305) -> ("MotorControlDevRef"=w315:T1)  [unwired: 7 in, 2 out]
            n167 = call <vilib>:"WPI_MotorControlSetOutput.vi"("Output"=w331, "MotorControlDevRef"=w333) -> ("MotorControlDevRef"=w329:T1)  [unwired: 7 in, 2 out]
            n168 = call <vilib>:"WPI_MotorControlSetOutput.vi"("Output"=w331, "MotorControlDevRef"=w332) -> ("MotorControlDevRef"=w330:T1)  [unwired: 7 in, 2 out]
            n169 = call <vilib>:"WPI_MotorControlSetOutput.vi"("Output"=w326, "MotorControlDevRef"=w328) -> ("MotorControlDevRef"=w325:T1)  [unwired: 7 in, 2 out]
            n170 = call <vilib>:"WPI_MotorControlSetOutput.vi"("Output"=w326, "MotorControlDevRef"=w327) -> ("MotorControlDevRef"=w320:T1)  [unwired: 7 in, 2 out]
            n171 = Greater Or Equal?(x=w324, y=14) -> (x >= y?=w321:bool)
            n172 = feedback #2() -> (w309:dbl)  [unwired: 1 in]
            n173 = Add(x=w309, y=w307) -> (x+y=w310:dbl)
            n174 = Subtract(x=w309, y=w307) -> (x-y=w308:dbl)
            n175 = In Range and Coerce(upper limit=w310, x=0.64 ("Output"), lower limit=w308) -> (coerced(x)=w311:dbl)  [unwired: 1 out]
            n176 = feedback-in #2(w311) -> ()
            n177 = call <vilib>:"WPI_MotorControlSetOutput.vi"("Output"=w311, "MotorControlDevRef"=w318) -> ("MotorControlDevRef"=w317:T1)  [unwired: 7 in, 2 out]
          }
          n178 = while {
            tunnel: [w302] -> _
            tunnel: [w301] -> _
            tunnel: [w299] -> _
            tunnel: [w294] -> _
            tunnel: [w292] -> _
            tunnel: [w291] -> _
            tunnel: [w290] -> _
            tunnel: [w289] -> _
            tunnel: w221 -> [w286]
            tunnel: w220 -> [w285]
            tunnel: w219 -> [w284]
            tunnel: w218 -> [w283]
            tunnel: w217 -> [w282]
            tunnel: w216 -> [w281]
            tunnel: w215 -> [w280]
            tunnel: w214 -> [w279]
            i -> [w296]
            stop <- w295 stop-if-true
            w293 = 1.0 ("Output")
            w300 = 0.0 ("Output")
            w303 = 0.0 ("Output")
            n179 = Increment(x=w296) -> (x+1=w298:i32)
            n180 = Wait (ms)(milliseconds to wait=u32 50) -> ()  [unwired: 1 out]
            n181 = call <vilib>:"WPI_MotorControlSetOutput.vi"("Output"=0.64, "MotorControlDevRef"=w283) -> ("MotorControlDevRef"=w292:T1)  [unwired: 7 in, 2 out]
            n182 = call <vilib>:"WPI_MotorControlSetOutput.vi"("Output"=w293, "MotorControlDevRef"=w286) -> ("MotorControlDevRef"=w289:T1)  [unwired: 7 in, 2 out]
            n183 = call <vilib>:"WPI_MotorControlSetOutput.vi"("Output"=w293, "MotorControlDevRef"=w285) -> ("MotorControlDevRef"=w291:T1)  [unwired: 7 in, 2 out]
            n184 = call <vilib>:"WPI_MotorControlSetOutput.vi"("Output"=w293, "MotorControlDevRef"=w284) -> ("MotorControlDevRef"=w290:T1)  [unwired: 7 in, 2 out]
            n185 = call <vilib>:"WPI_MotorControlSetOutput.vi"("Output"=w303, "MotorControlDevRef"=w282) -> ("MotorControlDevRef"=w301:T1)  [unwired: 7 in, 2 out]
            n186 = call <vilib>:"WPI_MotorControlSetOutput.vi"("Output"=w303, "MotorControlDevRef"=w281) -> ("MotorControlDevRef"=w302:T1)  [unwired: 7 in, 2 out]
            n187 = call <vilib>:"WPI_MotorControlSetOutput.vi"("Output"=w300, "MotorControlDevRef"=w280) -> ("MotorControlDevRef"=w299:T1)  [unwired: 7 in, 2 out]
            n188 = call <vilib>:"WPI_MotorControlSetOutput.vi"("Output"=w300, "MotorControlDevRef"=w279) -> ("MotorControlDevRef"=w294:T1)  [unwired: 7 in, 2 out]
            n189 = Greater Or Equal?(x=w298, y=14) -> (x >= y?=w295:bool)
          }
        }
        frame "Gear", Default {
          n190 = while {
            tunnel: [w552] -> w494
            tunnel: [w551] -> w495
            tunnel: [w550] -> w493
            tunnel: [w549] -> w492
            tunnel: [w546] -> w486
            tunnel: [w545] -> _
            tunnel: w478 -> [w544]
            tunnel: w479 -> [w543]
            tunnel: w480 -> [w542]
            tunnel: w477 -> [w541]
            tunnel: w481 -> [w540]
            stop <- w547 stop-if-true
            w545 = -96.0 ("y")
            w539 = -0.4 ("Output")
            w553 = -0.4 ("Output")
            n191 = call <vilib>:"WPI_EncoderGet.vi"("EncoderDevRef"=w541) -> ("Distance"=w548:dbl, "EncoderDevRef"=w546:T6)  [unwired: 5 in, 4 out]
            n192 = Wait (ms)(milliseconds to wait=u32 50) -> ()  [unwired: 1 out]
            n193 = Less Or Equal?(x=w548, y=w545) -> (x <= y?=w547:bool)
            n194 = call <vilib>:"WPI_MotorControlSetOutput.vi"("Output"=w553, "MotorControlDevRef"=w543) -> ("MotorControlDevRef"=w552:T1)  [unwired: 7 in, 2 out]
            n195 = call <vilib>:"WPI_MotorControlSetOutput.vi"("Output"=w553, "MotorControlDevRef"=w544) -> ("MotorControlDevRef"=w551:T1)  [unwired: 7 in, 2 out]
            n196 = call <vilib>:"WPI_MotorControlSetOutput.vi"("Output"=w539, "MotorControlDevRef"=w542) -> ("MotorControlDevRef"=w550:T1)  [unwired: 7 in, 2 out]
            n197 = call <vilib>:"WPI_MotorControlSetOutput.vi"("Output"=w539, "MotorControlDevRef"=w540) -> ("MotorControlDevRef"=w549:T1)  [unwired: 7 in, 2 out]
          }
          n198 = while {
            tunnel: w495 -> [w537]
            tunnel: w494 -> [w536]
            tunnel: [w534] -> w490
            tunnel: [w533] -> w491
            tunnel: w493 -> [w532]
            tunnel: w492 -> [w531]
            tunnel: [w529] -> w489
            tunnel: [w528] -> w488
            tunnel: [w525] -> w487
            tunnel: w486 -> [w524]
            tunnel: [w523] -> _
            stop <- w526 stop-if-true
            w523 = -120.0 ("y")
            w530 = 0.4 ("Output")
            w535 = -0.4 ("Output")
            n199 = call <vilib>:"WPI_EncoderGet.vi"("EncoderDevRef"=w524) -> ("Distance"=w527:dbl, "EncoderDevRef"=w525:T6)  [unwired: 5 in, 4 out]
            n200 = Wait (ms)(milliseconds to wait=u32 50) -> ()  [unwired: 1 out]
            n201 = Less Or Equal?(x=w527, y=w523) -> (x <= y?=w526:bool)
            n202 = call <vilib>:"WPI_MotorControlSetOutput.vi"("Output"=w535, "MotorControlDevRef"=w536) -> ("MotorControlDevRef"=w534:T1)  [unwired: 7 in, 2 out]
            n203 = call <vilib>:"WPI_MotorControlSetOutput.vi"("Output"=w535, "MotorControlDevRef"=w537) -> ("MotorControlDevRef"=w533:T1)  [unwired: 7 in, 2 out]
            n204 = call <vilib>:"WPI_MotorControlSetOutput.vi"("Output"=w530, "MotorControlDevRef"=w532) -> ("MotorControlDevRef"=w529:T1)  [unwired: 7 in, 2 out]
            n205 = call <vilib>:"WPI_MotorControlSetOutput.vi"("Output"=w530, "MotorControlDevRef"=w531) -> ("MotorControlDevRef"=w528:T1)  [unwired: 7 in, 2 out]
          }
          n206 = while {
            tunnel: w491 -> [w521]
            tunnel: w490 -> [w520]
            tunnel: [w518] -> w484
            tunnel: [w517] -> w485
            tunnel: w489 -> [w516]
            tunnel: w488 -> [w515]
            tunnel: [w513] -> w483
            tunnel: [w512] -> w482
            tunnel: [w508] -> _
            tunnel: w487 -> [w507]
            stop <- w509 stop-if-true
            w514 = -0.3 ("Output")
            w519 = -0.3 ("Output")
            n207 = call <vilib>:"WPI_EncoderGet.vi"("EncoderDevRef"=w507) -> ("Distance"=w511:dbl, "EncoderDevRef"=w508:T6)  [unwired: 5 in, 4 out]
            n208 = Wait (ms)(milliseconds to wait=u32 50) -> ()  [unwired: 1 out]
            n209 = call <vilib>:"WPI_MotorControlSetOutput.vi"("Output"=w519, "MotorControlDevRef"=w520) -> ("MotorControlDevRef"=w518:T1)  [unwired: 7 in, 2 out]
            n210 = call <vilib>:"WPI_MotorControlSetOutput.vi"("Output"=w519, "MotorControlDevRef"=w521) -> ("MotorControlDevRef"=w517:T1)  [unwired: 7 in, 2 out]
            n211 = call <vilib>:"WPI_MotorControlSetOutput.vi"("Output"=w514, "MotorControlDevRef"=w516) -> ("MotorControlDevRef"=w513:T1)  [unwired: 7 in, 2 out]
            n212 = call <vilib>:"WPI_MotorControlSetOutput.vi"("Output"=w514, "MotorControlDevRef"=w515) -> ("MotorControlDevRef"=w512:T1)  [unwired: 7 in, 2 out]
            n213 = Less Or Equal?(x=w511, y=-134.0) -> (x <= y?=w509:bool)
          }
          n214 = while {
            tunnel: w485 -> [w505]
            tunnel: w484 -> [w504]
            tunnel: w483 -> [w502]
            tunnel: w482 -> [w501]
            i -> [w499]
            stop <- w496 stop-if-true
            w500 = 0.0 ("Output")
            w503 = 0.0 ("Output")
            n215 = Increment(x=w499) -> (x+1=w498:i32)
            n216 = Wait (ms)(milliseconds to wait=u32 50) -> ()  [unwired: 1 out]
            n217 = Greater Or Equal?(x=w498, y=753000) -> (x >= y?=w496:bool)
            n218 = call <vilib>:"WPI_MotorControlSetOutput.vi"("Output"=w503, "MotorControlDevRef"=w504) -> ()  [unwired: 7 in, 3 out]
            n219 = call <vilib>:"WPI_MotorControlSetOutput.vi"("Output"=w503, "MotorControlDevRef"=w505) -> ()  [unwired: 7 in, 3 out]
            n220 = call <vilib>:"WPI_MotorControlSetOutput.vi"("Output"=w500, "MotorControlDevRef"=w502) -> ()  [unwired: 7 in, 3 out]
            n221 = call <vilib>:"WPI_MotorControlSetOutput.vi"("Output"=w500, "MotorControlDevRef"=w501) -> ()  [unwired: 7 in, 3 out]
          }
        }
      }
    }
    frame "Blue" {
      n222 = case shown="\"GearShoot\"" w564 {
        tunnel: w556 -> [_ _ w961]
        tunnel: w557 -> [w571 w756 w960]
        tunnel: w563 -> [w572 _ w959]
        tunnel: w562 -> [w570 w754 w958]
        tunnel: w561 -> [w569 w753 w957]
        tunnel: w560 -> [w568 w744 _]
        tunnel: w559 -> [w567 w745 _]
        tunnel: w555 -> [w566 w751 _]
        tunnel: w558 -> [w565 _ _]
        tunnel: w557 -> [_ w755 _]
        tunnel: w556 -> [_ w752 _]
        tunnel: w555 -> [_ w743 _]
        frame "Shoot" {
          n223 = while {
            tunnel: [w707] -> w603
            tunnel: [w706] -> w604
            tunnel: [w704] -> w602
            tunnel: [w703] -> w601
            tunnel: [w695] -> w600
            tunnel: [w694] -> w599
            tunnel: [w693] -> w598
            tunnel: [w692] -> w597
            tunnel: w572 -> [w687]
            tunnel: w571 -> [w686]
            tunnel: w570 -> [w685]
            tunnel: w569 -> [w684]
            tunnel: w568 -> [w683]
            tunnel: w567 -> [w682]
            tunnel: w566 -> [w681]
            tunnel: w565 -> [w680]
            i -> [w702]
            stop <- w699 stop-if-true
            w696 = 0.05
            w698 = 0.0 ("Output")
            w705 = 0.0 ("Output")
            w708 = 0.0 ("Output")
            n224 = Increment(x=w702) -> (x+1=w701:i32)
            n225 = Wait (ms)(milliseconds to wait=u32 50) -> ()  [unwired: 1 out]
            n226 = call <vilib>:"WPI_MotorControlSetOutput.vi"("Output"=w698, "MotorControlDevRef"=w682) -> ("MotorControlDevRef"=w693:T1)  [unwired: 7 in, 2 out]
            n227 = call <vilib>:"WPI_MotorControlSetOutput.vi"("Output"=w698, "MotorControlDevRef"=w681) -> ("MotorControlDevRef"=w692:T1)  [unwired: 7 in, 2 out]
            n228 = call <vilib>:"WPI_MotorControlSetOutput.vi"("Output"=w698, "MotorControlDevRef"=w683) -> ("MotorControlDevRef"=w694:T1)  [unwired: 7 in, 2 out]
            n229 = call <vilib>:"WPI_MotorControlSetOutput.vi"("Output"=w708, "MotorControlDevRef"=w685) -> ("MotorControlDevRef"=w706:T1)  [unwired: 7 in, 2 out]
            n230 = call <vilib>:"WPI_MotorControlSetOutput.vi"("Output"=w708, "MotorControlDevRef"=w684) -> ("MotorControlDevRef"=w707:T1)  [unwired: 7 in, 2 out]
            n231 = call <vilib>:"WPI_MotorControlSetOutput.vi"("Output"=w705, "MotorControlDevRef"=w687) -> ("MotorControlDevRef"=w704:T1)  [unwired: 7 in, 2 out]
            n232 = call <vilib>:"WPI_MotorControlSetOutput.vi"("Output"=w705, "MotorControlDevRef"=w686) -> ("MotorControlDevRef"=w703:T1)  [unwired: 7 in, 2 out]
            n233 = Greater Or Equal?(x=w701, y=45) -> (x >= y?=w699:bool)
            n234 = feedback #3() -> (w690:dbl)  [unwired: 1 in]
            n235 = Add(x=w690, y=w696) -> (x+y=w697:dbl)
            n236 = Subtract(x=w690, y=w696) -> (x-y=w688:dbl)
            n237 = In Range and Coerce(upper limit=w697, x=0.603 ("Output"), lower limit=w688) -> (coerced(x)=w691:dbl)  [unwired: 1 out]
            n238 = feedback-in #3(w691) -> ()
            n239 = call <vilib>:"WPI_MotorControlSetOutput.vi"("Output"=w691, "MotorControlDevRef"=w680) -> ("MotorControlDevRef"=w695:T1)  [unwired: 7 in, 2 out]
          }
          n240 = while {
            tunnel: [w732] -> w590
            tunnel: [w731] -> w589
            tunnel: [w729] -> w592
            tunnel: [w728] -> w591
            tunnel: w604 -> [w721]
            tunnel: w603 -> [w720]
            tunnel: w602 -> [w719]
            tunnel: w601 -> [w718]
            tunnel: w600 -> [w717]
            tunnel: w599 -> [w716]
            tunnel: w598 -> [w715]
            tunnel: w597 -> [w714]
            tunnel: [w713] -> w594
            tunnel: [w712] -> w593
            tunnel: [w711] -> w595
            tunnel: [w710] -> w596
            i -> [w727]
            stop <- w724 stop-if-true
            w723 = 1.0 ("Output")
            w730 = 0.0 ("Output")
            w733 = 0.0 ("Output")
            n241 = Increment(x=w727) -> (x+1=w726:i32)
            n242 = Wait (ms)(milliseconds to wait=u32 50) -> ()  [unwired: 1 out]
            n243 = call <vilib>:"WPI_MotorControlSetOutput.vi"("Output"=w723, "MotorControlDevRef"=w715) -> ("MotorControlDevRef"=w713:T1)  [unwired: 7 in, 2 out]
            n244 = call <vilib>:"WPI_MotorControlSetOutput.vi"("Output"=w723, "MotorControlDevRef"=w714) -> ("MotorControlDevRef"=w712:T1)  [unwired: 7 in, 2 out]
            n245 = call <vilib>:"WPI_MotorControlSetOutput.vi"("Output"=w723, "MotorControlDevRef"=w716) -> ("MotorControlDevRef"=w711:T1)  [unwired: 7 in, 2 out]
            n246 = call <vilib>:"WPI_MotorControlSetOutput.vi"("Output"=w733, "MotorControlDevRef"=w721) -> ("MotorControlDevRef"=w731:T1)  [unwired: 7 in, 2 out]
            n247 = call <vilib>:"WPI_MotorControlSetOutput.vi"("Output"=w733, "MotorControlDevRef"=w720) -> ("MotorControlDevRef"=w732:T1)  [unwired: 7 in, 2 out]
            n248 = call <vilib>:"WPI_MotorControlSetOutput.vi"("Output"=w730, "MotorControlDevRef"=w719) -> ("MotorControlDevRef"=w729:T1)  [unwired: 7 in, 2 out]
            n249 = call <vilib>:"WPI_MotorControlSetOutput.vi"("Output"=w730, "MotorControlDevRef"=w718) -> ("MotorControlDevRef"=w728:T1)  [unwired: 7 in, 2 out]
            n250 = call <vilib>:"WPI_MotorControlSetOutput.vi"("Output"=0.603, "MotorControlDevRef"=w717) -> ("MotorControlDevRef"=w710:T1)  [unwired: 7 in, 2 out]
            n251 = Greater Or Equal?(x=w726, y=140) -> (x >= y?=w724:bool)
          }
          n252 = while {
            tunnel: [w677] -> w582
            tunnel: [w676] -> w581
            tunnel: [w674] -> w584
            tunnel: [w673] -> w583
            tunnel: w589 -> [w666]
            tunnel: w592 -> [w665]
            tunnel: w591 -> [w664]
            tunnel: w596 -> [w663]
            tunnel: w595 -> [w662]
            tunnel: w594 -> [w661]
            tunnel: w593 -> [w660]
            tunnel: [w659] -> w586
            tunnel: [w658] -> w585
            tunnel: [w657] -> w587
            tunnel: [w656] -> w588
            tunnel: w590 -> [w655]
            i -> [w672]
            stop <- w669 stop-if-true
            w668 = 0.0 ("Output")
            w675 = -0.5 ("Output")
            w678 = 0.4 ("Output")
            n253 = Increment(x=w672) -> (x+1=w671:i32)
            n254 = Wait (ms)(milliseconds to wait=u32 50) -> ()  [unwired: 1 out]
            n255 = call <vilib>:"WPI_MotorControlSetOutput.vi"("Output"=w668, "MotorControlDevRef"=w661) -> ("MotorControlDevRef"=w659:T1)  [unwired: 7 in, 2 out]
            n256 = call <vilib>:"WPI_MotorControlSetOutput.vi"("Output"=w668, "MotorControlDevRef"=w660) -> ("MotorControlDevRef"=w658:T1)  [unwired: 7 in, 2 out]
            n257 = call <vilib>:"WPI_MotorControlSetOutput.vi"("Output"=w668, "MotorControlDevRef"=w662) -> ("MotorControlDevRef"=w657:T1)  [unwired: 7 in, 2 out]
            n258 = call <vilib>:"WPI_MotorControlSetOutput.vi"("Output"=w678, "MotorControlDevRef"=w666) -> ("MotorControlDevRef"=w676:T1)  [unwired: 7 in, 2 out]
            n259 = call <vilib>:"WPI_MotorControlSetOutput.vi"("Output"=w678, "MotorControlDevRef"=w655) -> ("MotorControlDevRef"=w677:T1)  [unwired: 7 in, 2 out]
            n260 = call <vilib>:"WPI_MotorControlSetOutput.vi"("Output"=w675, "MotorControlDevRef"=w665) -> ("MotorControlDevRef"=w674:T1)  [unwired: 7 in, 2 out]
            n261 = call <vilib>:"WPI_MotorControlSetOutput.vi"("Output"=w675, "MotorControlDevRef"=w664) -> ("MotorControlDevRef"=w673:T1)  [unwired: 7 in, 2 out]
            n262 = Greater Or Equal?(x=w671, y=40) -> (x >= y?=w669:bool)
            n263 = call <vilib>:"WPI_MotorControlSetOutput.vi"("Output"=0.0, "MotorControlDevRef"=w663) -> ("MotorControlDevRef"=w656:T1)  [unwired: 7 in, 2 out]
          }
          n264 = while {
            tunnel: [w652] -> w574
            tunnel: [w651] -> w573
            tunnel: [w649] -> w576
            tunnel: [w648] -> w575
            tunnel: w581 -> [w641]
            tunnel: w584 -> [w640]
            tunnel: w583 -> [w639]
            tunnel: w588 -> [w638]
            tunnel: w587 -> [w637]
            tunnel: w586 -> [w636]
            tunnel: w585 -> [w635]
            tunnel: [w634] -> w578
            tunnel: [w633] -> w577
            tunnel: [w632] -> w579
            tunnel: [w631] -> w580
            tunnel: w582 -> [w630]
            i -> [w647]
            stop <- w644 stop-if-true
            w643 = 0.0 ("Output")
            w650 = -0.4 ("Output")
            w653 = -0.4 ("Output")
            n265 = Increment(x=w647) -> (x+1=w646:i32)
            n266 = Wait (ms)(milliseconds to wait=u32 50) -> ()  [unwired: 1 out]
            n267 = call <vilib>:"WPI_MotorControlSetOutput.vi"("Output"=w643, "MotorControlDevRef"=w636) -> ("MotorControlDevRef"=w634:T1)  [unwired: 7 in, 2 out]
            n268 = call <vilib>:"WPI_MotorControlSetOutput.vi"("Output"=w643, "MotorControlDevRef"=w635) -> ("MotorControlDevRef"=w633:T1)  [unwired: 7 in, 2 out]
            n269 = call <vilib>:"WPI_MotorControlSetOutput.vi"("Output"=w643, "MotorControlDevRef"=w637) -> ("MotorControlDevRef"=w632:T1)  [unwired: 7 in, 2 out]
            n270 = call <vilib>:"WPI_MotorControlSetOutput.vi"("Output"=w653, "MotorControlDevRef"=w641) -> ("MotorControlDevRef"=w651:T1)  [unwired: 7 in, 2 out]
            n271 = call <vilib>:"WPI_MotorControlSetOutput.vi"("Output"=w653, "MotorControlDevRef"=w630) -> ("MotorControlDevRef"=w652:T1)  [unwired: 7 in, 2 out]
            n272 = call <vilib>:"WPI_MotorControlSetOutput.vi"("Output"=w650, "MotorControlDevRef"=w640) -> ("MotorControlDevRef"=w649:T1)  [unwired: 7 in, 2 out]
            n273 = call <vilib>:"WPI_MotorControlSetOutput.vi"("Output"=w650, "MotorControlDevRef"=w639) -> ("MotorControlDevRef"=w648:T1)  [unwired: 7 in, 2 out]
            n274 = Greater Or Equal?(x=w646, y=140) -> (x >= y?=w644:bool)
            n275 = call <vilib>:"WPI_MotorControlSetOutput.vi"("Output"=0.0, "MotorControlDevRef"=w638) -> ("MotorControlDevRef"=w631:T1)  [unwired: 7 in, 2 out]
          }
          n276 = while {
            tunnel: [w627] -> _
            tunnel: [w626] -> _
            tunnel: [w624] -> _
            tunnel: [w623] -> _
            tunnel: w573 -> [w616]
            tunnel: w576 -> [w605]
            tunnel: w575 -> [w615]
            tunnel: w580 -> [w614]
            tunnel: w579 -> [w613]
            tunnel: w578 -> [w612]
            tunnel: w577 -> [w611]
            tunnel: [w610] -> _
            tunnel: [w609] -> _
            tunnel: [w608] -> _
            tunnel: [w607] -> _
            tunnel: w574 -> [w606]
            tunnel: [w605] -> _
            i -> [w622]
            stop <- w619 stop-if-true
            w618 = 0.0 ("Output")
            w625 = 0.0 ("Output")
            w628 = 0.0 ("Output")
            n277 = Increment(x=w622) -> (x+1=w621:i32)
            n278 = Wait (ms)(milliseconds to wait=u32 50) -> ()  [unwired: 1 out]
            n279 = Greater Or Equal?(x=w621, y=753000) -> (x >= y?=w619:bool)
            n280 = call <vilib>:"WPI_MotorControlSetOutput.vi"("Output"=w618, "MotorControlDevRef"=w612) -> ("MotorControlDevRef"=w610:T1)  [unwired: 7 in, 2 out]
            n281 = call <vilib>:"WPI_MotorControlSetOutput.vi"("Output"=w618, "MotorControlDevRef"=w611) -> ("MotorControlDevRef"=w609:T1)  [unwired: 7 in, 2 out]
            n282 = call <vilib>:"WPI_MotorControlSetOutput.vi"("Output"=w618, "MotorControlDevRef"=w613) -> ("MotorControlDevRef"=w608:T1)  [unwired: 7 in, 2 out]
            n283 = call <vilib>:"WPI_MotorControlSetOutput.vi"("Output"=w628, "MotorControlDevRef"=w616) -> ("MotorControlDevRef"=w626:T1)  [unwired: 7 in, 2 out]
            n284 = call <vilib>:"WPI_MotorControlSetOutput.vi"("Output"=w628, "MotorControlDevRef"=w606) -> ("MotorControlDevRef"=w627:T1)  [unwired: 7 in, 2 out]
            n285 = call <vilib>:"WPI_MotorControlSetOutput.vi"("Output"=w625, "MotorControlDevRef"=w605) -> ("MotorControlDevRef"=w624:T1)  [unwired: 7 in, 2 out]
            n286 = call <vilib>:"WPI_MotorControlSetOutput.vi"("Output"=w625, "MotorControlDevRef"=w615) -> ("MotorControlDevRef"=w623:T1)  [unwired: 7 in, 2 out]
            n287 = call <vilib>:"WPI_MotorControlSetOutput.vi"("Output"=0.0, "MotorControlDevRef"=w614) -> ("MotorControlDevRef"=w607:T1)  [unwired: 7 in, 2 out]
          }
        }
        frame "GearShoot" {
          # "This tells you the driver position\nand alliance color"
          n288 = while {
            tunnel: [w954] -> w793
            tunnel: [w953] -> w794
            tunnel: [w951] -> w792
            tunnel: [w950] -> w791
            tunnel: [w947] -> w785
            tunnel: [w946] -> w765
            tunnel: w756 -> [w945]
            tunnel: w755 -> [w944]
            tunnel: w754 -> [w943]
            tunnel: w753 -> [w942]
            tunnel: w752 -> [w941]
            stop <- w948 stop-if-true
            w946 = -96.0 ("y")
            w952 = -0.4 ("Output")
            w955 = -0.4 ("Output")
            n289 = call <vilib>:"WPI_EncoderGet.vi"("EncoderDevRef"=w941) -> ("Distance"=w949:dbl, "EncoderDevRef"=w947:T6)  [unwired: 5 in, 4 out]
            n290 = Wait (ms)(milliseconds to wait=u32 50) -> ()  [unwired: 1 out]
            n291 = Less Or Equal?(x=w949, y=w946) -> (x <= y?=w948:bool)
            n292 = call <vilib>:"WPI_MotorControlSetOutput.vi"("Output"=w955, "MotorControlDevRef"=w943) -> ("MotorControlDevRef"=w953:T1)  [unwired: 7 in, 2 out]
            n293 = call <vilib>:"WPI_MotorControlSetOutput.vi"("Output"=w955, "MotorControlDevRef"=w942) -> ("MotorControlDevRef"=w954:T1)  [unwired: 7 in, 2 out]
            n294 = call <vilib>:"WPI_MotorControlSetOutput.vi"("Output"=w952, "MotorControlDevRef"=w945) -> ("MotorControlDevRef"=w950:T1)  [unwired: 7 in, 2 out]
            n295 = call <vilib>:"WPI_MotorControlSetOutput.vi"("Output"=w952, "MotorControlDevRef"=w944) -> ("MotorControlDevRef"=w951:T1)  [unwired: 7 in, 2 out]
          }
          n296 = while {
            tunnel: w794 -> [w939]
            tunnel: w793 -> [w938]
            tunnel: [w936] -> w789
            tunnel: [w935] -> w790
            tunnel: w792 -> [w934]
            tunnel: w791 -> [w933]
            tunnel: [w931] -> w788
            tunnel: [w930] -> w787
            tunnel: [w927] -> w786
            tunnel: w785 -> [w926]
            tunnel: [w925] -> w764
            stop <- w928 stop-if-true
            w925 = -120.0 ("y")
            w932 = 0.2 ("Output")
            w937 = -0.2 ("Output")
            n297 = call <vilib>:"WPI_EncoderGet.vi"("EncoderDevRef"=w926) -> ("Distance"=w929:dbl, "EncoderDevRef"=w927:T6)  [unwired: 5 in, 4 out]
            n298 = Wait (ms)(milliseconds to wait=u32 50) -> ()  [unwired: 1 out]
            n299 = Less Or Equal?(x=w929, y=w925) -> (x <= y?=w928:bool)
            n300 = call <vilib>:"WPI_MotorControlSetOutput.vi"("Output"=w937, "MotorControlDevRef"=w939) -> ("MotorControlDevRef"=w935:T1)  [unwired: 7 in, 2 out]
            n301 = call <vilib>:"WPI_MotorControlSetOutput.vi"("Output"=w937, "MotorControlDevRef"=w938) -> ("MotorControlDevRef"=w936:T1)  [unwired: 7 in, 2 out]
            n302 = call <vilib>:"WPI_MotorControlSetOutput.vi"("Output"=w932, "MotorControlDevRef"=w933) -> ("MotorControlDevRef"=w930:T1)  [unwired: 7 in, 2 out]
            n303 = call <vilib>:"WPI_MotorControlSetOutput.vi"("Output"=w932, "MotorControlDevRef"=w934) -> ("MotorControlDevRef"=w931:T1)  [unwired: 7 in, 2 out]
          }
          n304 = while {
            tunnel: w790 -> [w923]
            tunnel: w789 -> [w922]
            tunnel: [w920] -> w783
            tunnel: [w919] -> w784
            tunnel: w788 -> [w918]
            tunnel: w787 -> [w917]
            tunnel: [w915] -> w782
            tunnel: [w914] -> w781
            tunnel: [w910] -> w780
            tunnel: w786 -> [w909]
            stop <- w911 stop-if-true
            w916 = -0.3 ("Output")
            w921 = -0.3 ("Output")
            n305 = call <vilib>:"WPI_EncoderGet.vi"("EncoderDevRef"=w909) -> ("Distance"=w913:dbl, "EncoderDevRef"=w910:T6)  [unwired: 5 in, 4 out]
            n306 = Wait (ms)(milliseconds to wait=u32 50) -> ()  [unwired: 1 out]
            n307 = call <vilib>:"WPI_MotorControlSetOutput.vi"("Output"=w921, "MotorControlDevRef"=w923) -> ("MotorControlDevRef"=w919:T1)  [unwired: 7 in, 2 out]
            n308 = call <vilib>:"WPI_MotorControlSetOutput.vi"("Output"=w921, "MotorControlDevRef"=w922) -> ("MotorControlDevRef"=w920:T1)  [unwired: 7 in, 2 out]
            n309 = call <vilib>:"WPI_MotorControlSetOutput.vi"("Output"=w916, "MotorControlDevRef"=w917) -> ("MotorControlDevRef"=w914:T1)  [unwired: 7 in, 2 out]
            n310 = call <vilib>:"WPI_MotorControlSetOutput.vi"("Output"=w916, "MotorControlDevRef"=w918) -> ("MotorControlDevRef"=w915:T1)  [unwired: 7 in, 2 out]
            n311 = Less Or Equal?(x=w913, y=-134.0) -> (x <= y?=w911:bool)
          }
          n312 = Subtract(x=w765, y=w764) -> (x-y=w763:dbl)
          n313 = Divide(x=w763, y=4.0) -> (x/y=w761:dbl)
          n314 = while {
            tunnel: w784 -> [w907]
            tunnel: w783 -> [w906]
            tunnel: [w904] -> w778
            tunnel: [w903] -> w779
            tunnel: w782 -> [w902]
            tunnel: w781 -> [w901]
            tunnel: [w899] -> w777
            tunnel: [w898] -> w776
            i -> [w897]
            stop <- w894 stop-if-true
            w900 = 0.0 ("Output")
            w905 = 0.0 ("Output")
            n315 = Increment(x=w897) -> (x+1=w896:i32)
            n316 = Wait (ms)(milliseconds to wait=u32 50) -> ()  [unwired: 1 out]
            n317 = call <vilib>:"WPI_MotorControlSetOutput.vi"("Output"=w905, "MotorControlDevRef"=w907) -> ("MotorControlDevRef"=w903:T1)  [unwired: 7 in, 2 out]
            n318 = call <vilib>:"WPI_MotorControlSetOutput.vi"("Output"=w905, "MotorControlDevRef"=w906) -> ("MotorControlDevRef"=w904:T1)  [unwired: 7 in, 2 out]
            n319 = call <vilib>:"WPI_MotorControlSetOutput.vi"("Output"=w900, "MotorControlDevRef"=w901) -> ("MotorControlDevRef"=w898:T1)  [unwired: 7 in, 2 out]
            n320 = call <vilib>:"WPI_MotorControlSetOutput.vi"("Output"=w900, "MotorControlDevRef"=w902) -> ("MotorControlDevRef"=w899:T1)  [unwired: 7 in, 2 out]
            n321 = Greater Or Equal?(x=w896, y=120) -> (x >= y?=w894:bool)
          }
          n322 = while {
            tunnel: w779 -> [w892]
            tunnel: w778 -> [w891]
            tunnel: [w889] -> w774
            tunnel: [w888] -> w775
            tunnel: w777 -> [w887]
            tunnel: w776 -> [w886]
            tunnel: [w884] -> w773
            tunnel: [w883] -> w772
            tunnel: [w882] -> w771
            tunnel: w780 -> [w881]
            tunnel: [w878] -> w760
            stop <- w879 stop-if-true
            w878 = -82.0 ("y")
            w885 = 0.3 ("Output")
            w890 = 0.3 ("Output")
            n323 = call <vilib>:"WPI_EncoderGet.vi"("EncoderDevRef"=w881) -> ("Distance"=w880:dbl, "EncoderDevRef"=w882:T6)  [unwired: 5 in, 4 out]
            n324 = Wait (ms)(milliseconds to wait=u32 50) -> ()  [unwired: 1 out]
            n325 = Greater Or Equal?(x=w880, y=w878) -> (x >= y?=w879:bool)
            n326 = call <vilib>:"WPI_MotorControlSetOutput.vi"("Output"=w890, "MotorControlDevRef"=w892) -> ("MotorControlDevRef"=w888:T1)  [unwired: 7 in, 2 out]
            n327 = call <vilib>:"WPI_MotorControlSetOutput.vi"("Output"=w890, "MotorControlDevRef"=w891) -> ("MotorControlDevRef"=w889:T1)  [unwired: 7 in, 2 out]
            n328 = call <vilib>:"WPI_MotorControlSetOutput.vi"("Output"=w885, "MotorControlDevRef"=w886) -> ("MotorControlDevRef"=w883:T1)  [unwired: 7 in, 2 out]
            n329 = call <vilib>:"WPI_MotorControlSetOutput.vi"("Output"=w885, "MotorControlDevRef"=w887) -> ("MotorControlDevRef"=w884:T1)  [unwired: 7 in, 2 out]
          }
          n330 = Add(x=w761, y=w760) -> (x+y=w758:dbl)
          n331 = while {
            tunnel: w775 -> [w876]
            tunnel: w774 -> [w875]
            tunnel: [w873] -> w767
            tunnel: [w872] -> w766
            tunnel: w773 -> [w871]
            tunnel: w772 -> [w870]
            tunnel: [w868] -> w768
            tunnel: [w867] -> w769
            tunnel: [w866] -> w770
            tunnel: w771 -> [w865]
            tunnel: w758 -> [w864]
            stop <- w862 stop-if-true
            w869 = -0.3 ("Output")
            w874 = 0.3 ("Output")
            n332 = call <vilib>:"WPI_EncoderGet.vi"("EncoderDevRef"=w865) -> ("Distance"=w863:dbl, "EncoderDevRef"=w866:T6)  [unwired: 5 in, 4 out]
            n333 = Wait (ms)(milliseconds to wait=u32 50) -> ()  [unwired: 1 out]
            n334 = Greater Or Equal?(x=w863, y=w864) -> (x >= y?=w862:bool)
            n335 = call <vilib>:"WPI_MotorControlSetOutput.vi"("Output"=w874, "MotorControlDevRef"=w876) -> ("MotorControlDevRef"=w872:T1)  [unwired: 7 in, 2 out]
            n336 = call <vilib>:"WPI_MotorControlSetOutput.vi"("Output"=w874, "MotorControlDevRef"=w875) -> ("MotorControlDevRef"=w873:T1)  [unwired: 7 in, 2 out]
            n337 = call <vilib>:"WPI_MotorControlSetOutput.vi"("Output"=w869, "MotorControlDevRef"=w870) -> ("MotorControlDevRef"=w867:T1)  [unwired: 7 in, 2 out]
            n338 = call <vilib>:"WPI_MotorControlSetOutput.vi"("Output"=w869, "MotorControlDevRef"=w871) -> ("MotorControlDevRef"=w868:T1)  [unwired: 7 in, 2 out]
          }
          n339 = Add(x=17.0, y=w758) -> (x+y=w757:dbl)
          n340 = while {
            tunnel: w766 -> [w860]
            tunnel: w767 -> [w859]
            tunnel: [w857] -> w746
            tunnel: [w856] -> w747
            tunnel: w768 -> [w855]
            tunnel: w769 -> [w854]
            tunnel: [w852] -> w749
            tunnel: [w851] -> w748
            tunnel: [w850] -> w750
            tunnel: w770 -> [w849]
            tunnel: w757 -> [w846]
            stop <- w847 stop-if-true
            w853 = 0.3 ("Output")
            w858 = 0.3 ("Output")
            n341 = call <vilib>:"WPI_EncoderGet.vi"("EncoderDevRef"=w849) -> ("Distance"=w848:dbl, "EncoderDevRef"=w850:T6)  [unwired: 5 in, 4 out]
            n342 = Wait (ms)(milliseconds to wait=u32 50) -> ()  [unwired: 1 out]
            n343 = Greater Or Equal?(x=w848, y=w846) -> (x >= y?=w847:bool)
            n344 = call <vilib>:"WPI_MotorControlSetOutput.vi"("Output"=w858, "MotorControlDevRef"=w860) -> ("MotorControlDevRef"=w856:T1)  [unwired: 7 in, 2 out]
            n345 = call <vilib>:"WPI_MotorControlSetOutput.vi"("Output"=w858, "MotorControlDevRef"=w859) -> ("MotorControlDevRef"=w857:T1)  [unwired: 7 in, 2 out]
            n346 = call <vilib>:"WPI_MotorControlSetOutput.vi"("Output"=w853, "MotorControlDevRef"=w854) -> ("MotorControlDevRef"=w851:T1)  [unwired: 7 in, 2 out]
            n347 = call <vilib>:"WPI_MotorControlSetOutput.vi"("Output"=w853, "MotorControlDevRef"=w855) -> ("MotorControlDevRef"=w852:T1)  [unwired: 7 in, 2 out]
          }
          n348 = while {
            tunnel: w751 -> [w813]
            tunnel: w750 -> [_]
            tunnel: w749 -> [w812]
            tunnel: w748 -> [w811]
            tunnel: w747 -> [w810]
            tunnel: w746 -> [w809]
            tunnel: w745 -> [w808]
            tunnel: w744 -> [w807]
            tunnel: w743 -> [w806]
            tunnel: [w805] -> w742
            tunnel: [w804] -> w741
            tunnel: [w803] -> w740
            tunnel: [w802] -> w739
            tunnel: [w801] -> w738
            tunnel: [w800] -> w737
            tunnel: [w799] -> w736
            tunnel: [w798] -> w735
            i -> [w796]
            stop <- w795 stop-if-true
            w816 = 0.0753
            w820 = 0.0 ("Output")
            w822 = 0.0 ("Output")
            w823 = 0.0 ("Output")
            n349 = Increment(x=w796) -> (x+1=w797:i32)
            n350 = Wait (ms)(milliseconds to wait=u32 50) -> ()  [unwired: 1 out]
            n351 = call <vilib>:"WPI_MotorControlSetOutput.vi"("Output"=w820, "MotorControlDevRef"=w808) -> ("MotorControlDevRef"=w802:T1)  [unwired: 7 in, 2 out]
            n352 = call <vilib>:"WPI_MotorControlSetOutput.vi"("Output"=w820, "MotorControlDevRef"=w806) -> ("MotorControlDevRef"=w804:T1)  [unwired: 7 in, 2 out]
            n353 = call <vilib>:"WPI_MotorControlSetOutput.vi"("Output"=w820, "MotorControlDevRef"=w807) -> ("MotorControlDevRef"=w803:T1)  [unwired: 7 in, 2 out]
            n354 = call <vilib>:"WPI_MotorControlSetOutput.vi"("Output"=w823, "MotorControlDevRef"=w810) -> ("MotorControlDevRef"=w800:T1)  [unwired: 7 in, 2 out]
            n355 = call <vilib>:"WPI_MotorControlSetOutput.vi"("Output"=w823, "MotorControlDevRef"=w809) -> ("MotorControlDevRef"=w801:T1)  [unwired: 7 in, 2 out]
            n356 = call <vilib>:"WPI_MotorControlSetOutput.vi"("Output"=w822, "MotorControlDevRef"=w811) -> ("MotorControlDevRef"=w799:T1)  [unwired: 7 in, 2 out]
            n357 = call <vilib>:"WPI_MotorControlSetOutput.vi"("Output"=w822, "MotorControlDevRef"=w812) -> ("MotorControlDevRef"=w798:T1)  [unwired: 7 in, 2 out]
            n358 = Greater Or Equal?(x=w797, y=14) -> (x >= y?=w795:bool)
            n359 = feedback #4() -> (w815:dbl)  [unwired: 1 in]
            n360 = Add(x=w815, y=w816) -> (x+y=w817:dbl)
            n361 = Subtract(x=w815, y=w816) -> (x-y=w814:dbl)
            n362 = In Range and Coerce(upper limit=w817, x=0.64 ("Output"), lower limit=w814) -> (coerced(x)=w818:dbl)  [unwired: 1 out]
            n363 = feedback-in #4(w818) -> ()
            n364 = call <vilib>:"WPI_MotorControlSetOutput.vi"("Output"=w818, "MotorControlDevRef"=w813) -> ("MotorControlDevRef"=w805:T1)  [unwired: 7 in, 2 out]
          }
          n365 = while {
            tunnel: [w843] -> _
            tunnel: [w842] -> _
            tunnel: [w840] -> _
            tunnel: [w839] -> _
            tunnel: w742 -> [w832]
            tunnel: w741 -> [w831]
            tunnel: w740 -> [w830]
            tunnel: w739 -> [w829]
            tunnel: w738 -> [w828]
            tunnel: w737 -> [w827]
            tunnel: w736 -> [w826]
            tunnel: w735 -> [w825]
            i -> [w838]
            stop <- w835 stop-if-true
            w834 = 1.0 ("Output")
            w841 = 0.0 ("Output")
            w844 = 0.0 ("Output")
            n366 = Increment(x=w838) -> (x+1=w837:i32)
            n367 = call <vilib>:"WPI_MotorControlSetOutput.vi"("Output"=0.64, "MotorControlDevRef"=w832) -> ()  [unwired: 7 in, 3 out]
            n368 = Wait (ms)(milliseconds to wait=u32 50) -> ()  [unwired: 1 out]
            n369 = Greater Or Equal?(x=w837, y=753000) -> (x >= y?=w835:bool)
            n370 = call <vilib>:"WPI_MotorControlSetOutput.vi"("Output"=w834, "MotorControlDevRef"=w829) -> ()  [unwired: 7 in, 3 out]
            n371 = call <vilib>:"WPI_MotorControlSetOutput.vi"("Output"=w834, "MotorControlDevRef"=w831) -> ()  [unwired: 7 in, 3 out]
            n372 = call <vilib>:"WPI_MotorControlSetOutput.vi"("Output"=w834, "MotorControlDevRef"=w830) -> ()  [unwired: 7 in, 3 out]
            n373 = call <vilib>:"WPI_MotorControlSetOutput.vi"("Output"=w844, "MotorControlDevRef"=w827) -> ("MotorControlDevRef"=w842:T1)  [unwired: 7 in, 2 out]
            n374 = call <vilib>:"WPI_MotorControlSetOutput.vi"("Output"=w844, "MotorControlDevRef"=w828) -> ("MotorControlDevRef"=w843:T1)  [unwired: 7 in, 2 out]
            n375 = call <vilib>:"WPI_MotorControlSetOutput.vi"("Output"=w841, "MotorControlDevRef"=w826) -> ("MotorControlDevRef"=w839:T1)  [unwired: 7 in, 2 out]
            n376 = call <vilib>:"WPI_MotorControlSetOutput.vi"("Output"=w841, "MotorControlDevRef"=w825) -> ("MotorControlDevRef"=w840:T1)  [unwired: 7 in, 2 out]
          }
          n377 = call <vilib>:"WPI_DriverStationGet Alliance Info.vi"() -> ()  [unwired: 12 out]
        }
        frame "Gear", Default {
          n378 = while {
            tunnel: [w1032] -> w974
            tunnel: [w1031] -> w975
            tunnel: [w1030] -> w973
            tunnel: [w1029] -> w972
            tunnel: [w1026] -> w966
            tunnel: [w1025] -> _
            tunnel: [w1022] -> _
            tunnel: w960 -> [w1024]
            tunnel: w961 -> [w1022]
            tunnel: w959 -> [w1021]
            tunnel: w958 -> [w1020]
            tunnel: w957 -> [w1019]
            stop <- w1027 stop-if-true
            w1025 = -96.0 ("y")
            w1023 = -0.4 ("Output")
            w1033 = -0.4 ("Output")
            n379 = call <vilib>:"WPI_EncoderGet.vi"("EncoderDevRef"=w1022) -> ("Distance"=w1028:dbl, "EncoderDevRef"=w1026:T6)  [unwired: 5 in, 4 out]
            n380 = Wait (ms)(milliseconds to wait=u32 50) -> ()  [unwired: 1 out]
            n381 = Less Or Equal?(x=w1028, y=w1025) -> (x <= y?=w1027:bool)
            n382 = call <vilib>:"WPI_MotorControlSetOutput.vi"("Output"=w1033, "MotorControlDevRef"=w1020) -> ("MotorControlDevRef"=w1032:T1)  [unwired: 7 in, 2 out]
            n383 = call <vilib>:"WPI_MotorControlSetOutput.vi"("Output"=w1033, "MotorControlDevRef"=w1019) -> ("MotorControlDevRef"=w1031:T1)  [unwired: 7 in, 2 out]
            n384 = call <vilib>:"WPI_MotorControlSetOutput.vi"("Output"=w1023, "MotorControlDevRef"=w1021) -> ("MotorControlDevRef"=w1030:T1)  [unwired: 7 in, 2 out]
            n385 = call <vilib>:"WPI_MotorControlSetOutput.vi"("Output"=w1023, "MotorControlDevRef"=w1024) -> ("MotorControlDevRef"=w1029:T1)  [unwired: 7 in, 2 out]
          }
          n386 = while {
            tunnel: w975 -> [w1017]
            tunnel: w974 -> [w1016]
            tunnel: [w1014] -> w970
            tunnel: [w1013] -> w971
            tunnel: w973 -> [w1012]
            tunnel: w972 -> [w1011]
            tunnel: [w1009] -> w969
            tunnel: [w1008] -> w968
            tunnel: [w1005] -> w967
            tunnel: w966 -> [w1004]
            tunnel: [w1003] -> _
            stop <- w1006 stop-if-true
            w1003 = -120.0 ("y")
            w1010 = 0.4 ("Output")
            w1015 = -0.4 ("Output")
            n387 = call <vilib>:"WPI_EncoderGet.vi"("EncoderDevRef"=w1004) -> ("Distance"=w1007:dbl, "EncoderDevRef"=w1005:T6)  [unwired: 5 in, 4 out]
            n388 = Wait (ms)(milliseconds to wait=u32 50) -> ()  [unwired: 1 out]
            n389 = Less Or Equal?(x=w1007, y=w1003) -> (x <= y?=w1006:bool)
            n390 = call <vilib>:"WPI_MotorControlSetOutput.vi"("Output"=w1015, "MotorControlDevRef"=w1016) -> ("MotorControlDevRef"=w1014:T1)  [unwired: 7 in, 2 out]
            n391 = call <vilib>:"WPI_MotorControlSetOutput.vi"("Output"=w1015, "MotorControlDevRef"=w1017) -> ("MotorControlDevRef"=w1013:T1)  [unwired: 7 in, 2 out]
            n392 = call <vilib>:"WPI_MotorControlSetOutput.vi"("Output"=w1010, "MotorControlDevRef"=w1012) -> ("MotorControlDevRef"=w1009:T1)  [unwired: 7 in, 2 out]
            n393 = call <vilib>:"WPI_MotorControlSetOutput.vi"("Output"=w1010, "MotorControlDevRef"=w1011) -> ("MotorControlDevRef"=w1008:T1)  [unwired: 7 in, 2 out]
          }
          n394 = while {
            tunnel: w971 -> [w1001]
            tunnel: w970 -> [w1000]
            tunnel: [w998] -> w964
            tunnel: [w997] -> w965
            tunnel: w969 -> [w996]
            tunnel: w968 -> [w995]
            tunnel: [w993] -> w963
            tunnel: [w992] -> w962
            tunnel: [w988] -> _
            tunnel: w967 -> [w987]
            stop <- w989 stop-if-true
            w994 = -0.3 ("Output")
            w999 = -0.3 ("Output")
            n395 = call <vilib>:"WPI_EncoderGet.vi"("EncoderDevRef"=w987) -> ("Distance"=w991:dbl, "EncoderDevRef"=w988:T6)  [unwired: 5 in, 4 out]
            n396 = Wait (ms)(milliseconds to wait=u32 50) -> ()  [unwired: 1 out]
            n397 = call <vilib>:"WPI_MotorControlSetOutput.vi"("Output"=w999, "MotorControlDevRef"=w1000) -> ("MotorControlDevRef"=w998:T1)  [unwired: 7 in, 2 out]
            n398 = call <vilib>:"WPI_MotorControlSetOutput.vi"("Output"=w999, "MotorControlDevRef"=w1001) -> ("MotorControlDevRef"=w997:T1)  [unwired: 7 in, 2 out]
            n399 = call <vilib>:"WPI_MotorControlSetOutput.vi"("Output"=w994, "MotorControlDevRef"=w996) -> ("MotorControlDevRef"=w993:T1)  [unwired: 7 in, 2 out]
            n400 = call <vilib>:"WPI_MotorControlSetOutput.vi"("Output"=w994, "MotorControlDevRef"=w995) -> ("MotorControlDevRef"=w992:T1)  [unwired: 7 in, 2 out]
            n401 = Less Or Equal?(x=w991, y=-134.0) -> (x <= y?=w989:bool)
          }
          n402 = while {
            tunnel: w965 -> [w985]
            tunnel: w964 -> [w984]
            tunnel: w963 -> [w982]
            tunnel: w962 -> [w981]
            i -> [w979]
            stop <- w976 stop-if-true
            w980 = 0.0 ("Output")
            w983 = 0.0 ("Output")
            n403 = Increment(x=w979) -> (x+1=w978:i32)
            n404 = Wait (ms)(milliseconds to wait=u32 50) -> ()  [unwired: 1 out]
            n405 = Greater Or Equal?(x=w978, y=753000) -> (x >= y?=w976:bool)
            n406 = call <vilib>:"WPI_MotorControlSetOutput.vi"("Output"=w983, "MotorControlDevRef"=w984) -> ()  [unwired: 7 in, 3 out]
            n407 = call <vilib>:"WPI_MotorControlSetOutput.vi"("Output"=w983, "MotorControlDevRef"=w985) -> ()  [unwired: 7 in, 3 out]
            n408 = call <vilib>:"WPI_MotorControlSetOutput.vi"("Output"=w980, "MotorControlDevRef"=w982) -> ()  [unwired: 7 in, 3 out]
            n409 = call <vilib>:"WPI_MotorControlSetOutput.vi"("Output"=w980, "MotorControlDevRef"=w981) -> ()  [unwired: 7 in, 3 out]
          }
        }
      }
    }
  }
